vi "anschlüsse.vi"() -> ()   [LabVIEW 2010]
uses:
  <vilib>/numeric/LVNumericRepresentation.ctl
  <vilib>/Utility/miscctls.llb/LVPointTypeDef.ctl
panel:
  in  "poly2-Pfad":path
  in  "VI-Pfad":path
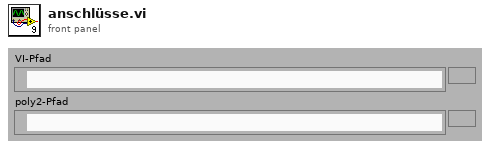
[diagram p1: front panel]
types:
  T1 = typedef "LVNumericRepresentation.ctl" = enum32{"Extended Precision", "Double Precision", "Single Precision", "Long", "Word", "Byte", "Unsigned Long", "Unsigned Word", "Unsigned Byte", "Complex Extended", "Complex Double", "Complex Single", "Quad", "Unsigned Quad", "Fixed-Point"}
  T2 = typedef "LVPointTypeDef.ctl" = cluster{"Horizontal":i16, "Vertical":i16}
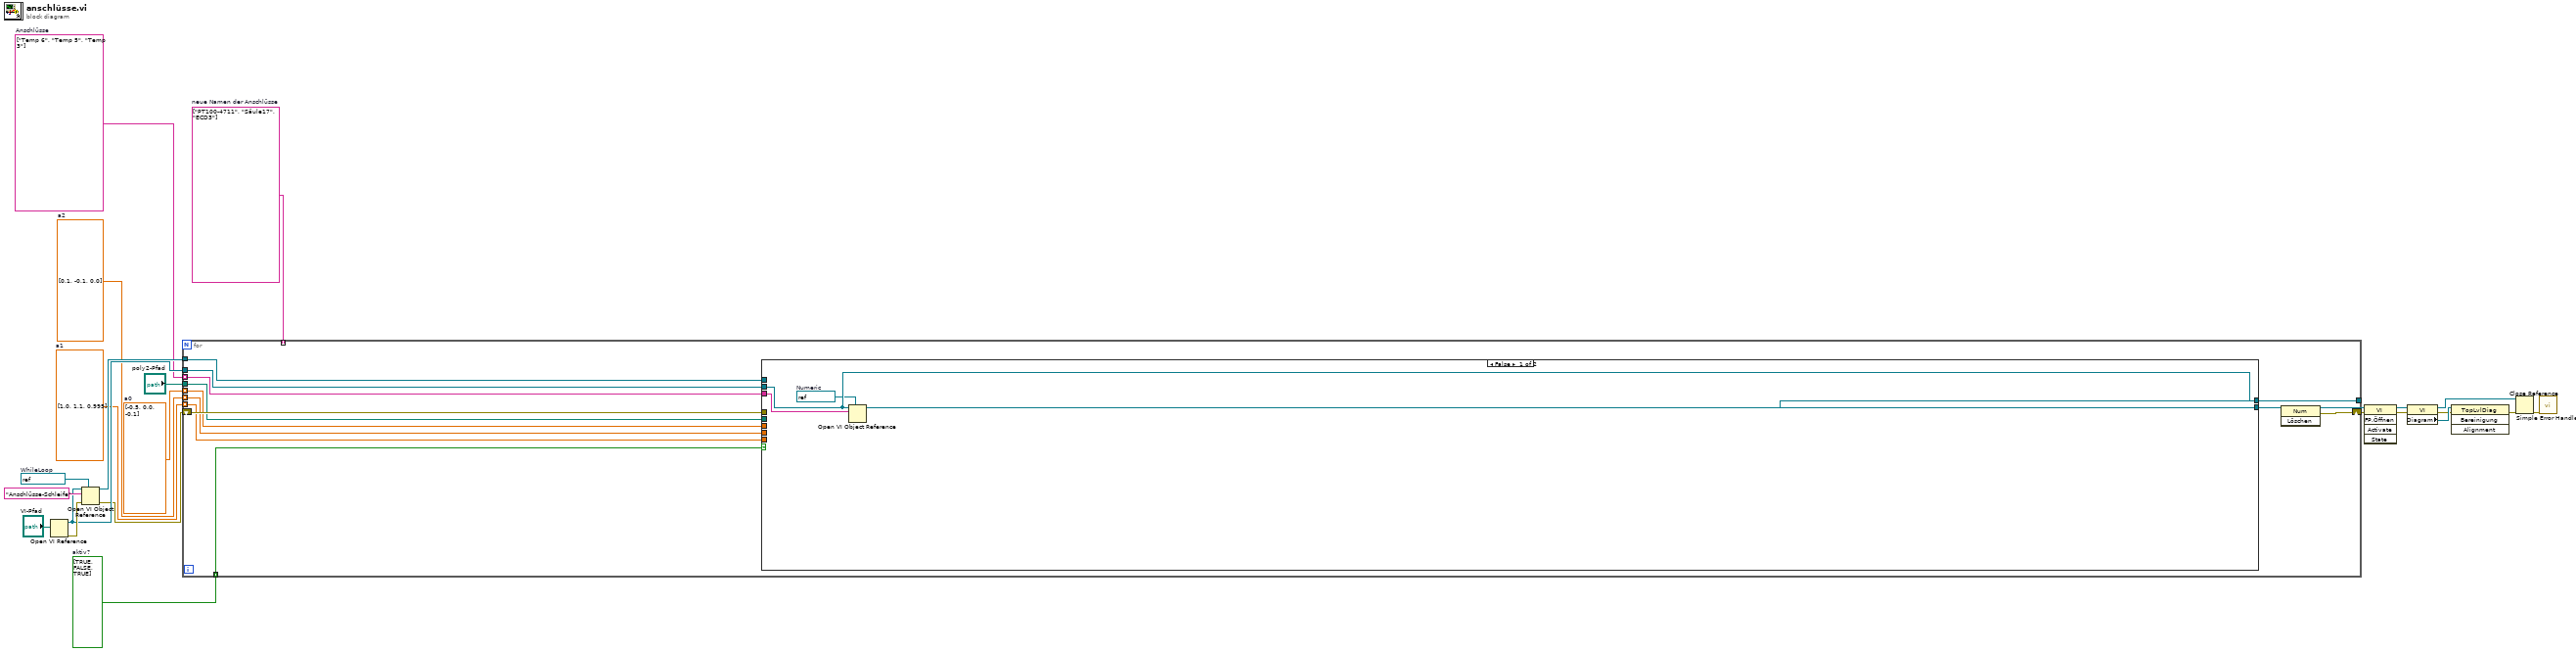
[diagram p0: block diagram]
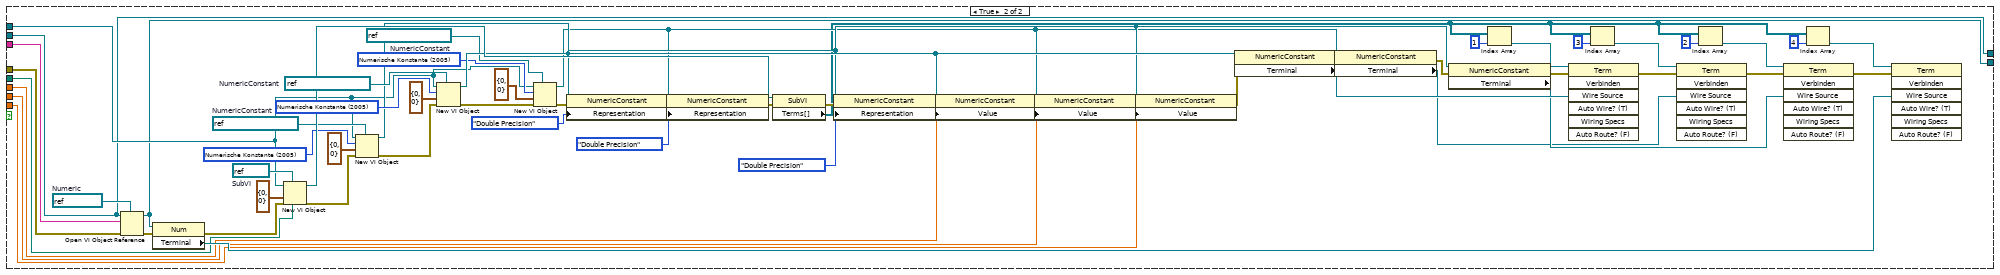
[diagram p2: hidden frame]
diagram:
  w1 = string[] ["PT100-4711", "Säule17", "ECD3"]  # neue Namen der Anschlüsse
  w2 = bool[] [TRUE, FALSE, TRUE]  # aktiv?
  w4 = dbl[] [-0.5, 0.0, -0.1]  # a0
  w5 = dbl[] [1.0, 1.1, 0.995]  # a1
  w6 = dbl[] [0.1, -0.1, 0.0]  # a2
  w15 = string[] ["Temp 6", "Temp 5", "Temp 3"]  # Anschlüsse
  w20 = refnum<vi> refnum  # WhileLoop
  n1 = Open VI Reference(vi path="VI-Pfad") -> (vi reference=w18:refnum<vi>, error out=w21:errorcluster)  [unwired: 5 in]
  n2 = Open VI Object Reference(7:w20, 8:w21, 10:"Anschlüsse-Schleife" ("Name/Position"), 11:w18) -> (0:w17:errorcluster, 3:w16:refnum<vi>)
  n3 = for {
    tunnel: w18 -> [w32]
    shift-right: [w35] -> w10
    shift-left: w17 -> [w34]
    tunnel: w16 -> [w33]
    tunnel: [w25] -> w3
    tunnel: w15 -> [w30] mode=indexing
    tunnel: "poly2-Pfad" -> [w31]
    tunnel: w6 -> [w28] mode=indexing
    tunnel: w5 -> [w27] mode=indexing
    tunnel: w4 -> [w29] mode=indexing
    tunnel: w2 -> [w24] mode=indexing
    tunnel: w1 -> [_] mode=indexing
    n4 = case shown="False" w24 {
      tunnel: w34 -> [_ w48]
      tunnel: w33 -> [_ w47]
      tunnel: w32 -> [w39 w40]
      tunnel: w31 -> [_ w46]
      tunnel: w30 -> [w38 w45]
      tunnel: w29 -> [_ w44]
      tunnel: w28 -> [_ w43]
      tunnel: w27 -> [_ w42]
      tunnel: [w36 w41] -> w26
      tunnel: [w39 w40] -> w25
      frame False {
        w37 = refnum<vi> refnum  # Numeric
        n5 = Open VI Object Reference(7:w37, 10:w38, 11:w39) -> (3:w36:refnum<vi>)  [unwired: 1 in, 1 out]
      }
      frame True {
        w77 = 2005 items=[".NET (Referenz)"=3441, ".NET-Container"=2125, "1D-Array dezimieren"=2046, "1D-Array durchsuchen"=1901, "1D-Array interpolieren"=1905, "1D-Array rotieren"=1906, "1D-Array sortieren"=1120, "1D-Array teilen"=1908, "1D-Array transponieren"=23068, "1D-Array umkehren"=1900, "1D-Arrays überführen"=2045, "2D-Array transponieren"=1902, "2D-Bild"=3508, "3-Zustands-Feld (System)"=21333, "3D-Bild"=23776, "Abbrechen-Schaltfläche (Modern)"=21739, "Abbrechen-Schaltfläche (System)"=3131, "Abgerundetes Rechteck"=3611, "Abgesenkter Kreis"=3604, "Abgesenkter Menüring"=3019, "Abgesenkter Rahmen (Modern)"=3607, "Abgesenkter Rahmen (System)"=3624, "Abgesenktes abgerundetes Rechteck"=3638, "Abgesenktes Dreieck (abwärts)"=3619, "Abgesenktes Dreieck (aufwärts)"=3618, "Abgesenktes Dreieck (links)"=3616, "Abgesenktes Dreieck (rechts)"=3617, "Abgesenktes Rechteck (dick)"=3635, "Abgesenktes Viereck"=3601, "Abgesenktes Viereck (abgerundet)"=3610, "Absoluter Wert"=1054, "ActiveX (Referenz)"=3410, "ActiveX-Container"=2072, "ActiveX-Objekt schließen"=8001, "ActiveX-Objekt öffnen"=8000, "Addieren"=1050, "AdrErstellen"=1967, "Agitator"=3831, "Aktivieren der Menüüberwachung"=9002, "AllSpoll"=1960, "Anzahl der Cache-Level"=24133, "Anzahl der Datensätze ermitteln"=8064, "Anzahl der Datensätze festlegen"=8075, "Applikationsreferenz"=3412, "Applikationsreferenz öffnen"=8012, "Arcuscosecans"=23050, "Arcuscosinus"=1207, "Arcuscotangens"=23052, "Arcussecans"=23051, "Arcussinus"=1206, "Arcustangens"=1208, "Arcustangens (2 Eingänge)"=1228, "Areacosecans"=23056, "Areacosinus Hyperbolicus"=1218, "Areacotangens"=23058, "Areasecans"=23057, "Areasinus Hyperbolicus"=1217, "Areatangens Hyperbolicus"=1219, "Array (Blockdiagrammkonstante)"=2070, "Array (Klassisch)"=3300, "Array (Modern)"=21608, "Array aus Strings nach Pfad"=1422, "Array erstellen"=2041, "Array indizieren"=2042, "Array initialisieren"=2053, "Array Interface Control"=23777, "Array nach Cluster"=1168, "Array nach Tabellen-String"=1540, "Array umformen"=2055, "Array wieder zusammensetzen"=2403, "Array zerlegen"=2412, "Array-Elemente addieren"=1903, "Array-Elemente multiplizieren"=1904, "Array-Größe"=1809, "Auf Aktion warten"=1722, "Auf Frontpanel-Aktivität warten"=1328, "Auf GPIB-RQS warten"=1952, "Auf Meldung mit Melderhistorie warten"=9131, "Auf Meldung von mehreren mit Melderhistorie warten"=9132, "Auf Meldung von mehreren warten"=9106, "Auf Meldung warten"=9105, "Auf nächste ganze Zahl runden"=1055, "Auf nächstgrößere Zahl runden"=1076, "Auf nächstkleinere Zahl runden"=1075, "Auf Occurrence warten"=1701, "Auf Stream-Status warten"=23809, "Auf Stream-Verknüpfung warten"=23799, "Aufruf über Referenz"=3901, "Aufrufkette"=1999, "Aufschlüsseln"=2048, "Aus Array entfernen"=3912, "Aus Binärdatei lesen"=8051, "Aus Textdatei lesen"=8070, "Aus XML zurückkonvertieren"=8401, "Ausdrucksknoten"=2201, "Austauscher"=3828, "Auswahlfeld (Klassisch)"=3117, "Auswahlfeld (Modern)"=21924, "Auswahlfeld (System)"=3132, "Auswahlfeld (System) 1"=21900, "Auswählen"=1516, "Avogadro-Konstante (1/mol)"=23520, "Basis des natürlichen Logarithmus"=23510, "Basiseinheiten umwandeln"=1079, "Baumstruktur (Klassisch)"=21819, "Baumstruktur (Modern)"=21793, "Baumstruktur (System)"=21794, "Bedingte Deaktivierungsstruktur"=2064, "Benutzerdef. Referenz"=3428, "Benutzerdef. Referenz-Tag (Blockdiagrammkonstante)"=3426, "Benutzerdef. Referenz-Tag (Klassisch)"=3429, "Benutzerdef. Referenz-Tag (Modern)"=21745, "Benutzerdef. Tag (Blockdiagrammkonstante)"=2114, "Benutzerdef. Tag (Klassisch)"=3329, "Benutzerdef. Tag (Modern)"=21749, "Benutzerdefiniertes Trace-Ereignis erzeugen"=2250, "Benutzerereignis erstellen"=2073, "Benutzerereignis erzeugen"=2074, "Benutzerereignis löschen"=2075, "Benutzerobjekt"=3506, "Berechtigungen ermitteln"=8065, "Berechtigungen festlegen"=8076, "Bereich"=2196, "Bereich sperren"=1411, "Beschriftete Schaltfläche (Rechteck)"=3123, "Beschriftete Schaltfläche (Rund)"=3122, "Beschriftete Schaltfläche (runde Ecken)"=3124, "Beschriftete Schaltfläche (runde Kanten)"=3125, "Beschriftung (Modern)"=21960, "Beschriftung (System)"=21961, "Bildlaufleiste (horizontal)"=21110, "Bildlaufleiste (vertikal)"=21111, "Bis zum nächsten Vielfachen von ms warten"=1327, "Bitpack nach Array"=3135, "Bluetooth - Auf Listener warten"=9147, "Bluetooth - Erkennung"=9152, "Bluetooth - Lesen"=9149, "Bluetooth - Listener erstellen"=9151, "Bluetooth - Netzwerkverbindung (Referenz)"=3468, "Bluetooth - Schreiben"=9150, "Bluetooth - Verbindung beenden"=9148, "Bluetooth - Verbindung herstellen"=9153, "Boolescher Wert nach (0,1)"=1167, "Boolesches Array nach Zahl"=1815, "Bruch-/Exponential-String nach Zahl"=1187, "Byte-Array nach String"=1609, "Bytes tauschen"=1162, "Bytestream-Datei (Referenz)"=3408, "Bündeln"=2049, "CAN-Kanal (Blockdiagrammkonstante)"=2124, "CAN-Kanal (Klassisch)"=3340, "CAN-Kanal (Modern)"=21817, "CAN-Kanal (System)"=21966, "CAN-Schnittstelle (Blockdiagrammkonstante)"=2123, "CAN-Schnittstelle (Klassisch)"=3339, "CAN-Schnittstelle (Modern)"=21815, "CAN-Schnittstelle (System)"=21964, "CAN-Task (Blockdiagrammkonstante)"=3471, "CAN-Task (Klassisch)"=3470, "CAN-Task (Modern)"=21789, "CAN-Task (System)"=21963, "Case-Struktur"=2001, "Cluster (Klassisch)"=3400, "Cluster (Modern)"=21607, "Cluster nach Array"=1169, "Cluster-Array erstellen"=2047, "Cluster-Array indizieren und bündeln"=2056, "Cluster-Konstante"=2071, "Code-Interface-Knoten"=2050, "Cosecans"=1204, "Cosecans Hyperbolicus"=23053, "Cosinus"=1201, "Cosinus Hyperbolicus"=1215, "Cotangens"=1205, "Cotangens Hyperbolicus"=23055, "CPU-Informationen"=24130, "DAQ-Kanal (Traditionell) (Blockdiagrammkonstante)"=2085, "DAQ-Kanal (Traditionell) (Klassisch)"=3320, "DAQ-Kanal (Traditionell) (Modern)"=21733, "DAQmx - Analog-Trigger-Quelle (Blockdiagrammkonstante)"=2119, "DAQmx - Analog-Trigger-Quelle (Klassisch)"=3336, "DAQmx - Analog-Trigger-Quelle (Modern)"=21774, "DAQmx - Analog-Trigger-Quelle (System)"=21951, "DAQmx - Globaler Kanal (Blockdiagrammkonstante)"=3430, "DAQmx - Globaler Kanal (Klassisch)"=3443, "DAQmx - Globaler Kanal (Modern)"=21770, "DAQmx - Globaler Kanal (System)"=21957, "DAQmx - Physikalischer Kanal (Blockdiagrammkonstante)"=2118, "DAQmx - Physikalischer Kanal (Klassisch)"=3335, "DAQmx - Physikalischer Kanal (Modern)"=21777, "DAQmx - Physikalischer Kanal (System)"=21954, "DAQmx-Anschluss (Blockdiagrammkonstante)"=2117, "DAQmx-Anschluss (Klassisch)"=3319, "DAQmx-Anschluss (Modern)"=21781, "DAQmx-Anschluss (System)"=21955, "DAQmx-Gerätename (Blockdiagrammkonstante)"=2093, "DAQmx-Gerätename (Klassisch)"=3318, "DAQmx-Gerätename (Modern)"=21773, "DAQmx-Gerätename (System)"=21950, "DAQmx-Skalierungsname (Blockdiagrammkonstante)"=2116, "DAQmx-Skalierungsname (Klassisch)"=3317, "DAQmx-Skalierungsname (Modern)"=21775, "DAQmx-Skalierungsname (System)"=21952, "DAQmx-Switch (Blockdiagrammkonstante)"=2121, "DAQmx-Switch (Klassisch)"=3337, "DAQmx-Switch (Modern)"=21776, "DAQmx-Switch (System)"=21953, "DAQmx-Task-Name (Blockdiagrammkonstante)"=3434, "DAQmx-Task-Name (Klassisch)"=3442, "DAQmx-Task-Name (Modern)"=21778, "DAQmx-Task-Name (System)"=21959, "DataSocket-Referenz"=3417, "DataSocket: Lesen"=1086, "DataSocket: Schließen"=1085, "DataSocket: Schreiben"=1087, "DataSocket: Öffnen"=1084, "Datei lesen"=1407, "Datei schließen"=8052, "Datei schließen (veraltet)"=1405, "Datei schreiben"=1408, "Datei öffnen"=1403, "Datei- und Programmtyp"=1434, "Datei- und Programmtyp ermitteln"=8066, "Datei- und Programmtyp festlegen"=8077, "Datei-/Verzeichnis-Info"=8082, "Datei-/Verzeichnis-Info (veraltet)"=1413, "Dateidialog"=8058, "Dateidialog (veraltet)"=8081, "Dateigröße ermitteln"=8063, "Dateigröße festlegen"=8074, "Dateipfad-Anzeigeelement (Klassisch)"=3204, "Dateipfad-Anzeigeelement (Modern)"=21731, "Dateipfad-Bedienelement (Klassisch)"=3203, "Dateipfad-Bedienelement (Modern)"=21730, "Dateipfad-Bedienelement (System)"=21922, "Dateiposition ermitteln"=8062, "Dateiposition festlegen"=8073, "Dateipuffer leeren"=8059, "Dateipuffer leeren (veraltet)"=1406, "Daten serialisieren"=1164, "Daten-Cache-Größe"=24132, "Datenprotokoll lesen"=8069, "Datenprotokoll schreiben"=8079, "Datenprotokolldatei (Referenz)"=3402, "Datenträger-Info"=1414, "Datenträger-Info lesen"=8067, "Datenwertreferenz löschen"=2409, "Datum-/Zeit-String lesen"=1600, "Datum/Zeit formatieren"=8100, "Datum/Zeit in Sekunden ermitteln"=1303, "Datum/Zeit nach Sekunden"=1308, "Dekrementieren"=1058, "DevClear"=1961, "DevClearList"=1962, "Dezimal-String nach Zahl"=1184, "Dezimalzeichen gleich?"=23064, "Dezimalziffer?"=1119, "Diagrammdeaktivierungsstruktur"=2054, "Dialogfeld mit einer Schaltfläche"=1340, "Dialogfeld mit zwei Schaltflächen"=1341, "Digitaldaten (Klassisch)"=3210, "Digitaldaten (Modern)"=21216, "Digitaler Signalverlaufsgraph (Klassisch)"=3511, "Digitaler Signalverlaufsgraph (Modern)"=21718, "Dividieren"=1053, "Dividieren (mit Fehleranschlüssen)"=3918, "Dlg Horiz. Bildlaufleiste"=21905, "Dlg Numerisch 1"=2100, "Dlg Numerisch 2"=3006, "Dlg String"=2110, "Dlg Vert. Bildlaufleiste"=21906, "Drehknopf (Klassisch)"=3005, "Drehknopf (Modern)"=21000, "Drehregler (Klassisch)"=3050, "Drehregler (Modern)"=21732, "Drehspulinstrument (Klassisch)"=3030, "Drehspulinstrument (Modern)"=21008, "Dreieck (abwärts)"=3623, "Dreieck (aufwärts)"=3622, "Dreieck (links)"=3620, "Dreieck (rechts)"=3621, "Dreiecksrelief (abwärts)"=3615, "Dreiecksrelief (aufwärts)"=3614, "Dreiecksrelief (links)"=3612, "Dreiecksrelief (rechts)"=3613, "Druckbar?"=1124, "Druckschalter"=21001, "Druckschalter (rechteckig)"=3119, "Druckschalter (rechteckig) (Profil)"=3113, "Druckschalter (rund)"=3118, "Druckschalter (rund) (Profil)"=3112, "Drucktank (flach)"=3075, "Drucktank (Klassisch)"=3070, "Drucktank (Modern)"=21751, "Drucktank (schattiert)"=21753, "Dynamische FPGA-Schnittstellen-Umwandlung"=5690, "Eigenschaftsknoten"=1920, "Ein Element aus Stream auslesen"=23797, "Ein Element in Stream schreiben"=23798, "Einfacher horiz. Schieber"=3003, "Einfacher String"=2115, "Einfacher vert. Schieber"=3002, "Einfaches numerisches Feld"=2900, "Einheit umrechnen"=2059, "Element am Anfang einfügen"=9129, "Element aus Queue entfernen"=9113, "Element einfügen"=9111, "Element einfügen (verlustbehaftet)"=9130, "Elementarladung (C)"=23517, "Elementreferenz"=3419, "Elternmethode aufrufen"=2354, "Empfangen"=1974, "Empfangsendpunkt für Netzwerk-Stream erstellen"=23811, "EnableLocal"=1963, "EnableRemote"=1964, "Enum (Klassisch)"=3023, "Enum (Modern)"=21605, "Enum (System)"=3062, "Enum-Konstante"=2090, "EOF"=1410, "Ereignis-Callback (Referenz)"=3435, "Ereignis-Callback registrieren"=2078, "Ereignisdatenknoten"=2102, "Ereignisregistrierung aufheben"=2076, "Ereignisstruktur"=2052, "Ersten String suchen"=1532, "Erster Aufruf?"=1083, "Exklusiv-NICHT-ODER"=1073, "Exklusiv-ODER"=1063, "Exponential"=1211, "Exponential (Arg) -1"=1222, "FALSE-Konstante"=2006, "Farbfeld"=3013, "Farbfeld mit dünnem Rahmen"=2905, "Farbfeld mit Rahmen (Klassisch)"=3008, "Farbfeld mit Rahmen (Modern)"=21019, "Farbfeldkonstante"=2120, "Farbiges Rechteck (Fehler?)"=3625, "Farbrampe"=3022, "Fehler zusammenfassen"=2147, "Fehler-Ringkonstante"=2039, "Festkomma in Integer umwandeln"=5566, "Festkomma-Überlaufzustand einschließen"=5564, "Festkomma-Überlaufzustand entfernen"=5563, "Festkomma-Überlaufzustand löschen"=5562, "Festkommakomponenten erfassen"=11163, "Festkommaüberlauf?"=5565, "FieldPoint-I/O-Kanal (Blockdiagrammkonstante)"=3440, "FieldPoint-I/O-Kanal (Klassisch)"=3439, "FieldPoint-I/O-Kanal (Modern)"=21784, "FIFO (Referenz)"=3474, "FindLstn"=1965, "FindRQS"=1966, "Flache Sequenzstruktur"=2069, "Fließkantenrelief (horizontal)"=3633, "Fließkantenrelief (vertikal)"=3634, "For-Schleife"=2002, "Formelknoten"=2004, "FPGA-Referenz nach Session"=2322, "Freie Beschriftung"=2321, "Frontpanel-Aktivität generieren"=1329, "Förderband"=3827, "Für Ereignisse registrieren"=2065, "Gabelung"=2194, "Gerät lesen"=1432, "Gerät schreiben"=1431, "Gerät öffnen"=1430, "Gerätereferenz"=3405, "Gerätsteuerung/Status"=1433, "Gestapelte Sequenzstruktur"=2000, "Gleich 0?"=1113, "Gleich?"=1102, "Globale Variable"=2060, "GPIB: Initialisierung"=1957, "GPIB: Lesen"=1951, "GPIB: Schreiben"=1950, "GPIB: Serielles Pollen"=1955, "GPIB: Status"=1959, "GPIB: Trigger"=1953, "GPIB: Verschiedenes"=1956, "GPIB: Warten"=1958, "GPIB: Zurücksetzen"=1954, "Grafikring (Klassisch)"=3015, "Grafikring (Modern)"=21602, "Grafikring (System)"=21925, "Gravitationskonstante (N m2/kg2)"=23519, "Größen-Handle"=1603, "Größer als 0?"=1117, "Größer oder gleich 0?"=1114, "Größer oder gleich?"=1103, "Größer?"=1110, "Heizkessel"=3829, "Hexadezimal-String nach Zahl"=1185, "Hexadezimalziffer?"=1123, "Hilfefenster steuern"=1353, "Hinzufügen (mit Fehleranschlüssen)"=3915, "Horiz. Linie"=3821, "Horiz. Rohrleitung (flach)"=3810, "Horiz. Rohrleitung (schattiert)"=3710, "Horiz. Rundbox"=3636, "Horizontaler Trennbalken (Klassisch)"=21863, "Horizontaler Trennbalken (System)"=21865, "ID des aktuellen Prozessors"=24131, "IMAQ-Session"=3415, "Immer kopieren"=2400, "Implikation"=1080, "In Array einfügen"=3911, "In Binärdatei schreiben"=8078, "In Datei formatieren"=2083, "In Datei suchen"=2082, "In Großbuchstaben"=1188, "In Kleinbuchstaben"=1189, "In OLE-Variant"=8002, "In String formatieren"=2081, "In String suchen"=2080, "In Textdatei schreiben"=8080, "In XML konvertieren"=8400, "Inkrementieren"=1057, "Inline-C-Knoten"=2104, "Inplace-Elementstruktur"=2360, "Integer in Festkomma umwandeln"=5567, "Intensitätsdiagramm (Klassisch)"=3509, "Intensitätsdiagramm (Modern)"=21719, "Intensitätsgraph (Klassisch)"=3510, "Intensitätsgraph (Modern)"=21720, "Intervall #1"=3073, "Intervall #2"=21755, "IP nach String"=1710, "IrDA-Netzwerkverbindung (Referenz)"=3450, "IrDA: Auf Listener warten"=9143, "IrDA: Geräte suchen"=9141, "IrDA: Lesen"=9145, "IrDA: Listener erzeugen"=9140, "IrDA: Schreiben"=9146, "IrDA: Verbindung herstellen"=9142, "IrDA: Verbindung schließen"=9144, "IVI Session löschen"=8103, "Kehrwert"=1059, "Kehrwert von e"=23511, "Kehrwert von Pi"=23507, "Kein Pfad (Konstante)"=23524, "Keine Referenz (Konstante)"=23526, "Keine Umgebungsvariable"=23527, "Keine Zahl/Kein Pfad/Keine Referenz?"=1128, "Kippschalter"=21002, "Kippschalter (vertikal)"=21740, "Klassenbezeichner-Konstante"=2094, "Kleiner als 0?"=1118, "Kleiner oder gleich 0?"=1115, "Kleiner oder gleich?"=1104, "Kleiner?"=1111, "Knoten zum Aufruf externer Bibliotheken"=2062, "Kombinationsfeld (Klassisch)"=3304, "Kombinationsfeld (Modern)"=21604, "Kombinationsfeld (System)"=21917, "Kombinationsfeldkonstante"=2088, "Komplex nach polar"=1045, "Komplex nach Re/Im"=1044, "Komplex-Konjugierte"=1048, "Kompressor"=3832, "Konstruktorknoten"=3904, "Kopieren"=8053, "Kopieren (veraltet)"=1416, "Kreis"=3605, "Kreisförmiges Relief"=3603, "Kreuzung"=2197, "LabVIEW beenden"=1352, "LabVIEW-Objekt"=3457, "Laufzeitklasse erhalten"=8018, "Leak Variant Value Reference"=2410, "LED (rechteckig) (Klassisch)"=3121, "LED (rechteckig) (Modern)"=21013, "LED (rund) (Klassisch)"=3120, "LED (rund) (Modern)"=21012, "LED-Schalter"=3116, "Leerer Pfad (Konstante)"=23523, "Leerer String (Konstante)"=23503, "Leerer String/Pfad?"=1112, "Leeres Array?"=23063, "Leuchte (rechteckig)"=3105, "Leuchte (rund)"=3104, "Lexikalische Klasse"=1126, "Lichtgeschwindigkeit im Vakuum (m/s)"=23518, "Linie (dick)"=3629, "Linie (dünn)"=3626, "Linie (vertieft) (System)"=3632, "Linie (vertieft, dick)"=3630, "Linie (vertieft, dünn)"=3627, "Linie mit Pfeil (dick)"=3631, "Linie mit Pfeil (dünn)"=3628, "Listenfeld (Klassisch)"=21806, "Listenfeld (Modern)"=21792, "Listenfeld (System)"=21805, "Listenfeldsymbol-Ringkonstante"=2038, "Logarithmus zur Basis 10"=1210, "Logarithmus zur Basis 10 von e"=23512, "Logarithmus zur Basis 2"=1225, "Logarithmus zur Basis x"=1224, "Logischer IVI-Name (Blockdiagrammkonstante)"=3420, "Logischer IVI-Name (Klassisch)"=3414, "Logischer IVI-Name (Modern)"=21736, "Logisches Verschieben"=1081, "Lokale Variable"=2061, "Löschen"=8056, "Löschen (veraltet)"=1417, "Mantisse und Exponent"=1150, "Maschinengenauigkeit"=23528, "MathScript-Aufruf über Referenzknoten"=3906, "MathScript-Knoten"=2357, "MATLAB-Skript"=9020, "Matrix entpacken"=23000, "Matrix erstellen"=8500, "Matrix transponieren"=8509, "Matrixdiagonale festlegen"=8504, "Matrixdiagonale lesen"=8501, "Matrixelemente festlegen"=8505, "Matrixelemente lesen"=8502, "Matrixgröße"=8507, "Matrixgröße ändern"=8508, "Max & Min"=1108, "Max. & Min. von Array"=1907, "Mehrere Elemente aus Stream auslesen"=23803, "Mehrere Elemente in Stream schreiben"=23804, "Mehrfacharithmetik"=2200, "Mehrsegmentrohr"=23780, "Mehrspaltiges Listenfeld (Klassisch)"=21799, "Mehrspaltiges Listenfeld (Modern)"=21791, "Mehrspaltiges Listenfeld (System)"=21798, "Melder anfordern"=9101, "Melder freigeben"=9102, "Melderreferenz"=3423, "Melderstatus lesen"=9103, "Meldung abbrechen"=9107, "Meldung senden"=9104, "Menü-Popup-Ring"=3017, "Menüauswahl abfragen"=9001, "Menüleiste des aktuellen VIs"=9000, "Menüpunkt-Info lesen"=9005, "Menüpunkte einfügen"=9003, "Menüpunkte löschen"=9004, "Menüpunkteinstellungen"=9006, "Menüreferenz"=3413, "Menüring (Klassisch)"=3018, "Menüring (Modern)"=21600, "Menüverknüpfung abfragen"=9007, "Messleiste (horizontal)"=21106, "Messleiste (vertikal)"=21107, "Methodenknoten"=3900, "Mischsignalgraph"=21721, "Mit Potenz von 2 multiplizieren"=1074, "Molare Gas-Konstante (J/(mol K))"=23522, "Motion-Ressource (Blockdiagrammkonstante)"=3449, "Motion-Ressource (Klassisch)"=3448, "Motion-Ressource (Modern)"=21787, "Motor (flach)"=3820, "Motor (schattiert)"=3720, "Multifrequenzstruktur"=2199, "Multiplizieren"=1052, "Multiplizieren (mit Fehleranschlüssen)"=3917, "Muster suchen"=1535, "Nach allgemeinerer Klasse"=8017, "Nach Byte-Integer"=1140, "Nach Festkomma"=5561, "Nach Fließkommawert (doppelte Genauigkeit)"=1147, "Nach Fließkommawert (einfache Genauigkeit)"=1146, "Nach Fließkommawert (erweitert)"=1149, "Nach Komplex (doppelte Genauigkeit)"=1152, "Nach Komplex (einfache Genauigkeit)"=1151, "Nach Komplex (höchste Genauigkeit)"=1154, "Nach links rotieren (mit Übertrag)"=1606, "Nach Long-Integer"=1142, "Nach Namen aufschlüsseln"=2058, "Nach Namen bündeln"=2057, "Nach Quad-Integer"=1155, "Nach rechts rotieren (mit Übertrag)"=1607, "Nach Sonden-String"=2413, "Nach spezifischerer Klasse"=8016, "Nach Variant"=8201, "Nach vorzeichenlosen Byte-Integer"=1143, "Nach vorzeichenlosen Long-Integer"=1145, "Nach vorzeichenlosen Quad-Integer"=1156, "Nach vorzeichenlosen Wort-Integer"=1144, "Nach Wert durchsuchen"=1534, "Nach Wort-Integer"=1141, "Nach Zeitstempel"=5560, "Natürlicher Logarithmus"=1209, "Natürlicher Logarithmus (Arg +1)"=1221, "Natürlicher Logarithmus von 10"=23513, "Natürlicher Logarithmus von 2"=23514, "Natürlicher Logarithmus von Pi"=23508, "Negativ unendlich"=23509, "Negieren"=1069, "Neue Datei"=1404, "Neue Datenwertreferenz"=2408, "Neue IVI-Session"=8102, "Neues Verzeichnis"=1402, "Neues VI"=8014, "Neues VI-Objekt"=8015, "NICHT"=1064, "Nicht darstellbares Zeichen?"=1125, "Nicht-ODER"=1072, "Nicht-UND"=1071, "Numerische Konstante"=2005, "Numerisches Anzeigeelement (Klassisch)"=3001, "Numerisches Anzeigeelement (Modern)"=21004, "Numerisches Bedienelement (Klassisch)"=3000, "Numerisches Bedienelement (Modern)"=21003, "Numerisches Bedienelement (System)"=21919, "Occurrence (Referenz)"=3406, "Occurrence erzeugen"=1700, "Occurrence festlegen"=1702, "ODER"=1062, "ODER (Array-Elemente)"=1910, "Offener Tank (flach) (Klassisch)"=21752, "Offener Tank (schattiert) (Klassisch)"=3074, "OK-Schaltfläche (Modern)"=21738, "OK-Schaltfläche (System)"=3130, "Oktal-String nach Zahl"=1186, "Oktalziffer?"=1129, "OLE-Variant"=3150, "Online-Hilfe steuern"=1355, "Optionsfeld (rechteckig)"=3107, "Optionsfeld (rund)"=3106, "Optionsfeld (System)"=3133, "Optionsfelder (Klassisch)"=22003, "Optionsfelder (Modern)"=22001, "Optionsfelder (System)"=22002, "Ordner anzeigen"=8083, "Ordner erstellen"=8055, "Paketmatrix"=23001, "PassControl"=1968, "Peek-Operation verarbeiten"=1604, "Pfad des aktuellen VIs"=1426, "Pfad erstellen"=1419, "Pfad nach Array aus Strings"=1423, "Pfad nach String"=1077, "Pfad zerlegen"=1420, "Pfadkonstante"=2009, "Pfadtyp"=1421, "Pfeil (Abwärts)"=3824, "Pfeil (aufwärts)"=3823, "Pfeil (links)"=3826, "Pfeil (rechts)"=3825, "Pi"=23504, "Pi geteilt durch 2"=23506, "Pi multipliziert mit 2"=23505, "PixMap"=3505, "PixMap (Warnung: gefährlich)"=3507, "Planck-Konstante (J/Hz)"=23516, "Plattform: Flache Rechteck-Schaltfläche"=3134, "Plugin-Steuerung"=21820, "Poke-Operation verarbeiten"=1605, "Polar nach komplex"=1047, "Polar nach Re/Im"=23061, "Position im Datenprotokoll ermitteln"=8061, "Position im Datenprotokoll festlegen"=8072, "Positiv unendlich"=23515, "Potenz von 10"=1212, "Potenz von 2"=1223, "PPoll"=1969, "PPollConfig"=1970, "PPollUnconfig"=1971, "Pulldown-Menüring"=3061, "Pumpe (links) (flach)"=3813, "Pumpe (links) (schattiert)"=3713, "Pumpe (rechts) (flach)"=3819, "Pumpe (rechts) (schattiert)"=3719, "Quadrat"=23059, "Quadratwurzel"=1060, "Queue anfordern"=9108, "Queue freigeben"=9109, "Queue leeren"=9114, "Queue-Referenz"=3424, "Queue-Status lesen"=9110, "Quotient und Rest"=1056, "Rahmen"=3608, "RcvRespMsg"=1972, "Re/Im nach komplex"=1046, "Re/Im nach polar"=23060, "ReadStatus"=1973, "ReceiveSetup"=1975, "Rechteck"=3602, "Rechteckschaltfläche"=3103, "Referenz nach Pfad"=1424, "Referenz nach Session"=2306, "Referenz schließen"=8011, "Regel- und Simulationsschleife"=2099, "Registerkartenelement (Klassisch)"=3330, "Registerkartenelement (Modern)"=3332, "Registerkartenelement (System)"=3331, "Registrierung für Sitzung entfernen"=2320, "Registrierungssession"=2319, "Reliefrahmen"=3606, "ResetSys"=1976, "Ressourcen-Index"=1088, "Rohrknie (links, abwärts) (flach)"=3811, "Rohrknie (links, abwärts) (schattiert)"=3711, "Rohrknie (links, aufwärts) (flach)"=3708, "Rohrknie (links, aufwärts) (flach) 1"=3808, "Rohrknie (rechts, abwärts) (flach)"=3817, "Rohrknie (rechts, abwärts) (schattiert)"=3717, "Rohrknie (rechts, aufwärts) (flach)"=3814, "Rohrknie (rechts, aufwärts) (schattiert)"=3714, "Rotationsverteiler"=3830, "Rotieren"=1082, "RT-FIFO erstellen"=24000, "RT-FIFO lesen"=24001, "RT-FIFO löschen"=24003, "RT-FIFO schreiben"=24002, "Rundinstrument (Klassisch)"=3040, "Rundinstrument (Modern)"=21009, "Rundschaltfläche"=3102, "Rydberg-Konstante (1/m)"=23521, "Rückkopplungsknoten"=2353, "Schalter (horizontal)"=3108, "Schalter (vertikal)"=3109, "Schaltfläche (rechteckig)"=3101, "Schaltfläche (rund)"=3100, "Schieber (horizontal) (Klassisch)"=3010, "Schieber (horizontal) (System)"=21904, "Schieber (horizontal, gefüllt) (Klassisch)"=3012, "Schieber (horizontal, gefüllt) (Modern)"=21100, "Schieber (vertikal) (System)"=21903, "Schieber (vertikal, gefüllt) (Klassisch)"=3009, "Schieber (vertikal, gefüllt) (Modern)"=21014, "Schieber mit Knopf (vertikal)"=3004, "Schieber mit Zeiger (horizontal) (Klassisch)"=3011, "Schieber mit Zeiger (horizontal) (Modern)"=21101, "Schieber mit Zeiger (horizontal) (System)"=21902, "Schieber mit Zeiger (vertikal) (Klassisch)"=3007, "Schieber mit Zeiger (vertikal) (Modern)"=21017, "Schieber mit Zeiger (vertikal) (System)"=21901, "Schiebeschalter"=21011, "Schiebeschalter (horizontal)"=3114, "Schiebeschalter (vertikal) (Klassisch)"=3115, "Schiebeschalter (vertikal) (Modern)"=21741, "Schwellwert (1D-Array)"=1909, "Secans"=1203, "Secans Hyperbolicus"=23054, "Sekunden nach Datum/Zeit"=1309, "SendCmds"=1978, "SendDataBytes"=1979, "Sendeendpunkt für Netzwerk-Stream erstellen"=23810, "Senden"=1977, "SendIFC"=1980, "SendList"=1981, "SendLLO"=1982, "SendSetup"=1983, "Serialisierte Daten nach Variant"=8202, "Serialisiertes benutzerdef. Referenz-Tag (Klassisch)"=3454, "Serialisiertes benutzerdef. Referenz-Tag (Modern)"=21747, "Session nach Referenz"=2307, "SetRWLS"=1984, "SetTimeOut"=1985, "Signale trennen"=2351, "Signale zusammenfassen"=2350, "Signalverlauf erstellen"=2066, "Signalverlaufsattribut entfernen"=8209, "Signalverlaufsattribut ermitteln"=8208, "Signalverlaufsattribut festlegen"=8207, "Signalverlaufsdiagramm"=21010, "Signalverlaufsdiagramm (Klassisch)"=3501, "Signalverlaufsdiagramm (Modern)"=21717, "Signalverlaufsgraph (Klassisch)"=3504, "Signalverlaufsgraph (Modern)"=21703, "Signalverlaufskomponenten lesen"=2067, "Sinc"=1227, "Sinus"=1200, "Sinus Hyperbolicus"=1214, "Sinus und Cosinus"=1220, "Speicherfreigabe anfordern"=1610, "Standardverzeichnis"=1427, "Statische VI-Referenz"=2084, "Status des Hilfefensters lesen"=1354, "Stopp"=1350, "Stopp-Schaltfläche"=21230, "Stopp-Schaltfläche (rechteckig)"=3128, "Stopp-Schaltfläche (rund)"=3127, "Stream beenden"=23807, "Stream erstellen"=23796, "Stream leeren"=23808, "Stream prüfen und verknüpfen"=23805, "Stream starten"=23806, "Stream verknüpfen"=23793, "Stream-Endpunkt entfernen"=23794, "Stream-Verknüpfung aufheben"=23795, "String deserialisieren"=1165, "String durchsuchen und teilen"=1538, "String nach Byte-Array"=1608, "String nach IP"=1711, "String nach Pfad"=1078, "String nach Token durchsuchen"=8101, "String nach Umgebungsvariable"=1830, "String rotieren"=1536, "String suchen und ersetzen"=3914, "String umkehren"=1537, "String-Anzeigeelement (Klassisch)"=3201, "String-Anzeigeelement (Modern)"=21702, "String-Array indizieren"=1531, "String-Bedienelement (Klassisch)"=3200, "String-Bedienelement (Modern)"=21701, "String-Bedienelement (System)"=21920, "String-Konstante"=2007, "String-Länge"=1502, "Stringarray sortieren"=23065, "Strings verknüpfen"=2040, "Subtrahieren"=1051, "Subtrahieren (mit Fehleranschlüssen)"=3916, "Suchen"=1409, "T-Stück (abwärts) (flach)"=3818, "T-Stück (abwärts) (schattiert)"=3718, "T-Stück (aufwärts) (flach)"=3812, "T-Stück (aufwärts) (schattiert)"=3712, "T-Stück (links) (flach)"=3809, "T-Stück (links) (schattiert)"=3709, "T-Stück (rechts) (flach)"=3815, "T-Stück (rechts) (schattiert)"=3715, "Tabelle (Klassisch)"=21796, "Tabelle (Modern)"=21790, "Tabelle (System)"=21797, "Tabellen-String nach Array"=1539, "Tabulatorkonstante"=23502, "Tag-Attributring"=2063, "Tangens"=1202, "Tangens Hyperbolicus"=1216, "Tank (horizontal)"=3071, "Tank (Klassisch)"=3020, "Tank (Modern)"=21006, "TCP-Netzwerkverbindung (Referenz)"=3407, "TCP: Auf Listener warten"=1712, "TCP: Lesen"=1716, "TCP: Lesen (Flex.)"=1720, "TCP: Lesen (Strings)"=1718, "TCP: Listener erstellen"=1717, "TCP: Schreiben"=1714, "TCP: Schreiben (Flex.)"=1721, "TCP: Schreiben (Strings)"=1719, "TCP: Verbindung herstellen"=1715, "TCP: Verbindung schließen"=1713, "TDMS Close"=24113, "TDMS Defragment"=24119, "TDMS Flush"=24117, "TDMS Get Properties"=24115, "TDMS List Contents"=24116, "TDMS Open"=24112, "TDMS Read"=24111, "TDMS Refnum To File ID"=24120, "TDMS Set Properties"=24114, "TDMS Write"=24110, "TDMS Write IP"=24118, "TDMS: Datei"=3477, "Teil-Array"=2044, "Teil-Array ersetzen"=3910, "Teil-String"=1503, "Teil-String ersetzen"=3913, "Temporäres Verzeichnis"=1435, "TestSRQ"=1986, "TestSys"=1987, "Text nach UTF-8"=23066, "Text- & Grafikring (Klassisch)"=3016, "Text- & Grafikring (Modern)"=21603, "Text-Schaltfläche"=21015, "Textring (Blockdiagrammkonstante)"=2008, "Textring (Klassisch)"=3014, "Textring (Modern)"=21601, "Textring (System)"=3060, "Thermometer (Klassisch)"=3021, "Thermometer (Modern)"=21007, "Timer-Wert (ms)"=1300, "Trennbalken (horizontal)"=21861, "Trennbalken (vertikal)"=21860, "Trennschalter"=21020, "Trichter 1"=21754, "Trichter 2"=3072, "Trigger"=1988, "TriggerList"=1989, "TRUE/FALSE-String anhängen"=1511, "TRUE/FALSE-String suchen"=1533, "Typ erzwingen"=2402, "Typumwandlung"=1166, "UDP-Netzwerkverbindung (Referenz)"=3418, "UDP: Lesen"=1724, "UDP: Multicast öffnen"=1727, "UDP: Schließen"=1726, "UDP: Schreiben"=1725, "UDP: Öffnen"=1723, "Umgebungsvariable"=23778, "Umgebungsvariable nach String"=1831, "Umgebungsvariablenelement (Klassisch)"=3472, "Umgebungsvariablenelement (Modern)"=21814, "Umgebungsvariablenkonstante"=3473, "Umschalter (horizontal) (Klassisch)"=3110, "Umschalter (horizontal) (Modern)"=21700, "Umschalter (vertikal) (Klassisch)"=3111, "Umschalter (vertikal) (Modern)"=21005, "Unbitpack von Array"=3136, "UND"=1061, "UND (Array-Elemente)"=1911, "Ungleich 0?"=1116, "Ungleich?"=1105, "Unleak Variant Value Reference"=2411, "Untermatrix festlegen"=8506, "Untermatrix lesen"=8503, "Unterpanel"=21810, "Unterpanel (klassisch)"=21811, "Unterpanel (System)"=21823, "UTF-8 nach Text"=23067, "Variable auslesen (mit Timeout)"=23786, "Variable direkt lesen"=23785, "Variable direkt schreiben"=23788, "Variable lesen"=23781, "Variable lesen (Scan)"=23784, "Variable schreiben"=23782, "Variable schreiben (mit Timeout)"=23789, "Variable schreiben (Scan)"=23787, "Variablen-Container suchen"=23802, "Variablenklassenbezeichner-Konstante"=2106, "Variablenkonfiguration"=3475, "Variablenname (Konstante)"=3478, "Variablenverbindung beenden"=23783, "Variablenverbindung herstellen"=23779, "Variablenverbindung herstellen und prüfen"=23790, "Variablenverbindung im Hintergrund herstellen"=23791, "Variant"=3310, "Variant nach Daten"=8003, "Variant nach serialisierte Daten"=8203, "Variant wieder zusammensetzen (Warnung: gefährlich)"=2405, "Variant zerlegen"=2404, "Variantattribut entfernen"=8206, "Variantattribut ermitteln"=8205, "Variantattribut festlegen"=8204, "Vektorwerte austauschen"=1912, "Ventil (Abwärtsbogen) (flach)"=3707, "Ventil (Abwärtsbogen) (schattiert)"=21767, "Ventil (Abwärtsbogen) (Umriss)"=3807, "Ventil (Aufwärtsbogen) (flach)"=3703, "Ventil (Aufwärtsbogen) (schattiert)"=21763, "Ventil (Aufwärtsbogen) (Umriss)"=3803, "Ventil (Linksbogen) (flach)"=3701, "Ventil (Linksbogen) (schattiert)"=21761, "Ventil (Linksbogen) (Umriss)"=3801, "Ventil (Rechtsbogen) (flach)"=3705, "Ventil (Rechtsbogen) (schattiert)"=21765, "Ventil (Rechtsbogen) (Umriss)"=3805, "Ventil (rechtwinklig, abwärts) (flach)"=3706, "Ventil (rechtwinklig, abwärts) (schattiert)"=21766, "Ventil (rechtwinklig, abwärts) (Umriss)"=3806, "Ventil (rechtwinklig, aufwärts) (flach)"=3702, "Ventil (rechtwinklig, aufwärts) (schattiert)"=3802, "Ventil (rechtwinklig, aufwärts) (Umriss)"=21762, "Ventil (rechtwinklig, links) (flach)"=3700, "Ventil (rechtwinklig, links) (schattiert)"=21760, "Ventil (rechtwinklig, links) (Umriss)"=3800, "Ventil (rechtwinklig, rechts) (flach)"=3704, "Ventil (rechtwinklig, rechts) (schattiert)"=21764, "Ventil (rechtwinklig, rechts) (Umriss)"=3804, "Ventil prüfen"=3833, "Vereinigung"=2195, "Verlaufsanzeige (horizontal) (Modern)"=21102, "Verlaufsanzeige (horizontal) (System)"=21910, "Verlaufsanzeige (vertikal) (Modern)"=21104, "Verlaufsanzeige (vertikal) (System)"=21909, "Verschieben"=8068, "Verschieben (veraltet)"=1415, "Verschobene Daten ermitteln"=9154, "Vert. Linie"=3822, "Vert. Rohrleitung (flach)"=3816, "Vert. Rohrleitung (schattiert)"=3716, "Vertikaler Trennbalken (Klassisch)"=21862, "Vertikaler Trennbalken (System)"=21864, "Verzeichnis auflisten"=1418, "VI-Bibliothek"=1425, "VI-Objektreferenz öffnen"=8013, "VI-Referenz"=3422, "VI-Referenz öffnen"=8010, "VI-Server-Referenz"=2091, "Viereckiges Relief (Klassisch)"=3600, "Viereckiges Relief (Modern)"=3637, "Viereckiges Relief (runde Ecken)"=3609, "VISA-Referenz nach Session"=2300, "VISA-Ressourcenname"=3421, "VISA-Ressourcenname (Klassisch)"=3409, "VISA-Ressourcenname (Modern)"=21737, "VISA: Adresse freigeben"=1933, "VISA: Adresse zuweisen"=1932, "VISA: Auf Ereignis warten"=1943, "VISA: Bereich lesen (16)"=1948, "VISA: Bereich lesen (32)"=1991, "VISA: Bereich lesen (64)"=2144, "VISA: Bereich lesen (8)"=1946, "VISA: Bereich schreiben (16)"=1949, "VISA: Bereich schreiben (32)"=1992, "VISA: Bereich schreiben (64)"=2145, "VISA: Bereich schreiben (8)"=1947, "VISA: Ereignis aktivieren"=1942, "VISA: Ereignis deaktivieren"=1940, "VISA: Ereignis verwerfen"=1941, "VISA: GPIB sendet IFC"=2318, "VISA: GPIB steuert ATN"=2316, "VISA: GPIB steuert REN"=2304, "VISA: GPIB-Befehl"=2315, "VISA: GPIB-Durchgangssteuerung"=2317, "VISA: Hilfssignal anfordern"=2310, "VISA: I/O-Puffer entleeren"=2302, "VISA: I/O-Puffergröße festlegen"=2301, "VISA: In Datei lesen"=2313, "VISA: Interrupt anfordern"=2309, "VISA: Lesen"=1925, "VISA: Peek (16)"=1934, "VISA: Peek (32)"=1995, "VISA: Peek (64)"=2142, "VISA: Peek (8)"=1938, "VISA: Poke (16)"=1935, "VISA: Poke (32)"=1996, "VISA: Poke (64)"=2143, "VISA: Poke (8)"=1939, "VISA: Ressource suchen"=1923, "VISA: Schließen"=1922, "VISA: Schreiben"=1926, "VISA: Speicher freigeben"=1998, "VISA: Speicher reservieren"=1997, "VISA: Speicher reservieren (Ex)"=2146, "VISA: Sperre aufheben"=1994, "VISA: Sperren"=1993, "VISA: Statusinformation"=1924, "VISA: STB lesen"=1928, "VISA: Trigger freigeben"=2312, "VISA: Trigger freigeben 1"=1929, "VISA: Trigger zuweisen"=2311, "VISA: USB-Steuerung (Ausgang)"=2087, "VISA: USB-Steuerung (Eingang)"=2086, "VISA: Verschieben"=2303, "VISA: Von Datei schreiben"=2314, "VISA: VXI-Befehl oder -Abfrage"=2305, "VISA: Wert lesen (16)"=1930, "VISA: Wert lesen (32)"=1944, "VISA: Wert lesen (64)"=2140, "VISA: Wert lesen (8)"=1936, "VISA: Wert schreiben (16)"=1931, "VISA: Wert schreiben (32)"=1945, "VISA: Wert schreiben (64)"=2141, "VISA: Wert schreiben (8)"=1937, "VISA: Zurücksetzen"=1927, "VISA: Öffnen"=2308, "VISA: Öffnen (alt)"=1921, "Vorschau für Queue-Element"=9112, "Vorzeichen"=1049, "Wagenrücklauf-Konstante"=23500, "WaitSRQ"=1990, "Warten (ms)"=1302, "Wert formatieren"=1512, "Werte austauschen"=2401, "Wertebereich prüfen und erzwingen"=1127, "While-Schleife 1"=2003, "While-Schleife 2"=2352, "Words tauschen"=1163, "X hoch Y"=1213, "XY-Graph (Klassisch)"=3500, "XY-Graph (Modern)"=21716, "Y-te Wurzel von X"=23062, "Zahl nach boolesches Array"=1814, "Zahl nach Hexadezimal-String"=1181, "Zahl nach Oktal-String"=1182, "Zahl nach String (Dezimaldarstellung)"=1180, "Zahl nach String (Exponentialdarstellung)"=1505, "Zahl nach String (Fließkommadarstellung)"=1506, "Zahl nach String (Technische Notation)"=1183, "Zahl teilen"=1170, "Zahlen verbinden"=1171, "Zeile auswählen"=1510, "Zeilenende-Konstante"=23525, "Zeilenvorschub-Konstante"=23501, "Zeitgesteuerte Schleife"=5570, "Zeitgesteuerte Sequenz"=5573, "Zeitstempel (Blockdiagrammkonstante)"=2068, "Zeitstempel-Anzeigeelement (Klassisch)"=5556, "Zeitstempel-Anzeigeelement (Modern)"=21914, "Zeitstempel-Bedienelement (Klassisch)"=5555, "Zeitstempel-Bedienelement (modern)"=21913, "Zeitstempel-Bedienelement (System)"=21967, "ZerlegenGesperrteDatenWertRef"=2406, "Zufallszahl (0-1)"=1070, "Zugriff verweigern"=8057, "Zugriffsrechte"=1412, "ZusammensetzenSperreAufhebenDatenWertRef (Warnung: gefährlich)"=2407, "Zustand"=2198, "Zustandsdiagramm"=2051, "Öffnen/Erstellen/Ersetzen einer Datei"=8050, "Öffnen/Erstellen/Ersetzen einer Protokolldatei"=8054]
        w76 = refnum<vi> refnum  # NumericConstant
        w71 = 2005 items=[".NET (Referenz)"=3441, ".NET-Container"=2125, "1D-Array dezimieren"=2046, "1D-Array durchsuchen"=1901, "1D-Array interpolieren"=1905, "1D-Array rotieren"=1906, "1D-Array sortieren"=1120, "1D-Array teilen"=1908, "1D-Array transponieren"=23068, "1D-Array umkehren"=1900, "1D-Arrays überführen"=2045, "2D-Array transponieren"=1902, "2D-Bild"=3508, "3-Zustands-Feld (System)"=21333, "3D-Bild"=23776, "Abbrechen-Schaltfläche (Modern)"=21739, "Abbrechen-Schaltfläche (System)"=3131, "Abgerundetes Rechteck"=3611, "Abgesenkter Kreis"=3604, "Abgesenkter Menüring"=3019, "Abgesenkter Rahmen (Modern)"=3607, "Abgesenkter Rahmen (System)"=3624, "Abgesenktes abgerundetes Rechteck"=3638, "Abgesenktes Dreieck (abwärts)"=3619, "Abgesenktes Dreieck (aufwärts)"=3618, "Abgesenktes Dreieck (links)"=3616, "Abgesenktes Dreieck (rechts)"=3617, "Abgesenktes Rechteck (dick)"=3635, "Abgesenktes Viereck"=3601, "Abgesenktes Viereck (abgerundet)"=3610, "Absoluter Wert"=1054, "ActiveX (Referenz)"=3410, "ActiveX-Container"=2072, "ActiveX-Objekt schließen"=8001, "ActiveX-Objekt öffnen"=8000, "Addieren"=1050, "AdrErstellen"=1967, "Agitator"=3831, "Aktivieren der Menüüberwachung"=9002, "AllSpoll"=1960, "Anzahl der Cache-Level"=24133, "Anzahl der Datensätze ermitteln"=8064, "Anzahl der Datensätze festlegen"=8075, "Applikationsreferenz"=3412, "Applikationsreferenz öffnen"=8012, "Arcuscosecans"=23050, "Arcuscosinus"=1207, "Arcuscotangens"=23052, "Arcussecans"=23051, "Arcussinus"=1206, "Arcustangens"=1208, "Arcustangens (2 Eingänge)"=1228, "Areacosecans"=23056, "Areacosinus Hyperbolicus"=1218, "Areacotangens"=23058, "Areasecans"=23057, "Areasinus Hyperbolicus"=1217, "Areatangens Hyperbolicus"=1219, "Array (Blockdiagrammkonstante)"=2070, "Array (Klassisch)"=3300, "Array (Modern)"=21608, "Array aus Strings nach Pfad"=1422, "Array erstellen"=2041, "Array indizieren"=2042, "Array initialisieren"=2053, "Array Interface Control"=23777, "Array nach Cluster"=1168, "Array nach Tabellen-String"=1540, "Array umformen"=2055, "Array wieder zusammensetzen"=2403, "Array zerlegen"=2412, "Array-Elemente addieren"=1903, "Array-Elemente multiplizieren"=1904, "Array-Größe"=1809, "Auf Aktion warten"=1722, "Auf Frontpanel-Aktivität warten"=1328, "Auf GPIB-RQS warten"=1952, "Auf Meldung mit Melderhistorie warten"=9131, "Auf Meldung von mehreren mit Melderhistorie warten"=9132, "Auf Meldung von mehreren warten"=9106, "Auf Meldung warten"=9105, "Auf nächste ganze Zahl runden"=1055, "Auf nächstgrößere Zahl runden"=1076, "Auf nächstkleinere Zahl runden"=1075, "Auf Occurrence warten"=1701, "Auf Stream-Status warten"=23809, "Auf Stream-Verknüpfung warten"=23799, "Aufruf über Referenz"=3901, "Aufrufkette"=1999, "Aufschlüsseln"=2048, "Aus Array entfernen"=3912, "Aus Binärdatei lesen"=8051, "Aus Textdatei lesen"=8070, "Aus XML zurückkonvertieren"=8401, "Ausdrucksknoten"=2201, "Austauscher"=3828, "Auswahlfeld (Klassisch)"=3117, "Auswahlfeld (Modern)"=21924, "Auswahlfeld (System)"=3132, "Auswahlfeld (System) 1"=21900, "Auswählen"=1516, "Avogadro-Konstante (1/mol)"=23520, "Basis des natürlichen Logarithmus"=23510, "Basiseinheiten umwandeln"=1079, "Baumstruktur (Klassisch)"=21819, "Baumstruktur (Modern)"=21793, "Baumstruktur (System)"=21794, "Bedingte Deaktivierungsstruktur"=2064, "Benutzerdef. Referenz"=3428, "Benutzerdef. Referenz-Tag (Blockdiagrammkonstante)"=3426, "Benutzerdef. Referenz-Tag (Klassisch)"=3429, "Benutzerdef. Referenz-Tag (Modern)"=21745, "Benutzerdef. Tag (Blockdiagrammkonstante)"=2114, "Benutzerdef. Tag (Klassisch)"=3329, "Benutzerdef. Tag (Modern)"=21749, "Benutzerdefiniertes Trace-Ereignis erzeugen"=2250, "Benutzerereignis erstellen"=2073, "Benutzerereignis erzeugen"=2074, "Benutzerereignis löschen"=2075, "Benutzerobjekt"=3506, "Berechtigungen ermitteln"=8065, "Berechtigungen festlegen"=8076, "Bereich"=2196, "Bereich sperren"=1411, "Beschriftete Schaltfläche (Rechteck)"=3123, "Beschriftete Schaltfläche (Rund)"=3122, "Beschriftete Schaltfläche (runde Ecken)"=3124, "Beschriftete Schaltfläche (runde Kanten)"=3125, "Beschriftung (Modern)"=21960, "Beschriftung (System)"=21961, "Bildlaufleiste (horizontal)"=21110, "Bildlaufleiste (vertikal)"=21111, "Bis zum nächsten Vielfachen von ms warten"=1327, "Bitpack nach Array"=3135, "Bluetooth - Auf Listener warten"=9147, "Bluetooth - Erkennung"=9152, "Bluetooth - Lesen"=9149, "Bluetooth - Listener erstellen"=9151, "Bluetooth - Netzwerkverbindung (Referenz)"=3468, "Bluetooth - Schreiben"=9150, "Bluetooth - Verbindung beenden"=9148, "Bluetooth - Verbindung herstellen"=9153, "Boolescher Wert nach (0,1)"=1167, "Boolesches Array nach Zahl"=1815, "Bruch-/Exponential-String nach Zahl"=1187, "Byte-Array nach String"=1609, "Bytes tauschen"=1162, "Bytestream-Datei (Referenz)"=3408, "Bündeln"=2049, "CAN-Kanal (Blockdiagrammkonstante)"=2124, "CAN-Kanal (Klassisch)"=3340, "CAN-Kanal (Modern)"=21817, "CAN-Kanal (System)"=21966, "CAN-Schnittstelle (Blockdiagrammkonstante)"=2123, "CAN-Schnittstelle (Klassisch)"=3339, "CAN-Schnittstelle (Modern)"=21815, "CAN-Schnittstelle (System)"=21964, "CAN-Task (Blockdiagrammkonstante)"=3471, "CAN-Task (Klassisch)"=3470, "CAN-Task (Modern)"=21789, "CAN-Task (System)"=21963, "Case-Struktur"=2001, "Cluster (Klassisch)"=3400, "Cluster (Modern)"=21607, "Cluster nach Array"=1169, "Cluster-Array erstellen"=2047, "Cluster-Array indizieren und bündeln"=2056, "Cluster-Konstante"=2071, "Code-Interface-Knoten"=2050, "Cosecans"=1204, "Cosecans Hyperbolicus"=23053, "Cosinus"=1201, "Cosinus Hyperbolicus"=1215, "Cotangens"=1205, "Cotangens Hyperbolicus"=23055, "CPU-Informationen"=24130, "DAQ-Kanal (Traditionell) (Blockdiagrammkonstante)"=2085, "DAQ-Kanal (Traditionell) (Klassisch)"=3320, "DAQ-Kanal (Traditionell) (Modern)"=21733, "DAQmx - Analog-Trigger-Quelle (Blockdiagrammkonstante)"=2119, "DAQmx - Analog-Trigger-Quelle (Klassisch)"=3336, "DAQmx - Analog-Trigger-Quelle (Modern)"=21774, "DAQmx - Analog-Trigger-Quelle (System)"=21951, "DAQmx - Globaler Kanal (Blockdiagrammkonstante)"=3430, "DAQmx - Globaler Kanal (Klassisch)"=3443, "DAQmx - Globaler Kanal (Modern)"=21770, "DAQmx - Globaler Kanal (System)"=21957, "DAQmx - Physikalischer Kanal (Blockdiagrammkonstante)"=2118, "DAQmx - Physikalischer Kanal (Klassisch)"=3335, "DAQmx - Physikalischer Kanal (Modern)"=21777, "DAQmx - Physikalischer Kanal (System)"=21954, "DAQmx-Anschluss (Blockdiagrammkonstante)"=2117, "DAQmx-Anschluss (Klassisch)"=3319, "DAQmx-Anschluss (Modern)"=21781, "DAQmx-Anschluss (System)"=21955, "DAQmx-Gerätename (Blockdiagrammkonstante)"=2093, "DAQmx-Gerätename (Klassisch)"=3318, "DAQmx-Gerätename (Modern)"=21773, "DAQmx-Gerätename (System)"=21950, "DAQmx-Skalierungsname (Blockdiagrammkonstante)"=2116, "DAQmx-Skalierungsname (Klassisch)"=3317, "DAQmx-Skalierungsname (Modern)"=21775, "DAQmx-Skalierungsname (System)"=21952, "DAQmx-Switch (Blockdiagrammkonstante)"=2121, "DAQmx-Switch (Klassisch)"=3337, "DAQmx-Switch (Modern)"=21776, "DAQmx-Switch (System)"=21953, "DAQmx-Task-Name (Blockdiagrammkonstante)"=3434, "DAQmx-Task-Name (Klassisch)"=3442, "DAQmx-Task-Name (Modern)"=21778, "DAQmx-Task-Name (System)"=21959, "DataSocket-Referenz"=3417, "DataSocket: Lesen"=1086, "DataSocket: Schließen"=1085, "DataSocket: Schreiben"=1087, "DataSocket: Öffnen"=1084, "Datei lesen"=1407, "Datei schließen"=8052, "Datei schließen (veraltet)"=1405, "Datei schreiben"=1408, "Datei öffnen"=1403, "Datei- und Programmtyp"=1434, "Datei- und Programmtyp ermitteln"=8066, "Datei- und Programmtyp festlegen"=8077, "Datei-/Verzeichnis-Info"=8082, "Datei-/Verzeichnis-Info (veraltet)"=1413, "Dateidialog"=8058, "Dateidialog (veraltet)"=8081, "Dateigröße ermitteln"=8063, "Dateigröße festlegen"=8074, "Dateipfad-Anzeigeelement (Klassisch)"=3204, "Dateipfad-Anzeigeelement (Modern)"=21731, "Dateipfad-Bedienelement (Klassisch)"=3203, "Dateipfad-Bedienelement (Modern)"=21730, "Dateipfad-Bedienelement (System)"=21922, "Dateiposition ermitteln"=8062, "Dateiposition festlegen"=8073, "Dateipuffer leeren"=8059, "Dateipuffer leeren (veraltet)"=1406, "Daten serialisieren"=1164, "Daten-Cache-Größe"=24132, "Datenprotokoll lesen"=8069, "Datenprotokoll schreiben"=8079, "Datenprotokolldatei (Referenz)"=3402, "Datenträger-Info"=1414, "Datenträger-Info lesen"=8067, "Datenwertreferenz löschen"=2409, "Datum-/Zeit-String lesen"=1600, "Datum/Zeit formatieren"=8100, "Datum/Zeit in Sekunden ermitteln"=1303, "Datum/Zeit nach Sekunden"=1308, "Dekrementieren"=1058, "DevClear"=1961, "DevClearList"=1962, "Dezimal-String nach Zahl"=1184, "Dezimalzeichen gleich?"=23064, "Dezimalziffer?"=1119, "Diagrammdeaktivierungsstruktur"=2054, "Dialogfeld mit einer Schaltfläche"=1340, "Dialogfeld mit zwei Schaltflächen"=1341, "Digitaldaten (Klassisch)"=3210, "Digitaldaten (Modern)"=21216, "Digitaler Signalverlaufsgraph (Klassisch)"=3511, "Digitaler Signalverlaufsgraph (Modern)"=21718, "Dividieren"=1053, "Dividieren (mit Fehleranschlüssen)"=3918, "Dlg Horiz. Bildlaufleiste"=21905, "Dlg Numerisch 1"=2100, "Dlg Numerisch 2"=3006, "Dlg String"=2110, "Dlg Vert. Bildlaufleiste"=21906, "Drehknopf (Klassisch)"=3005, "Drehknopf (Modern)"=21000, "Drehregler (Klassisch)"=3050, "Drehregler (Modern)"=21732, "Drehspulinstrument (Klassisch)"=3030, "Drehspulinstrument (Modern)"=21008, "Dreieck (abwärts)"=3623, "Dreieck (aufwärts)"=3622, "Dreieck (links)"=3620, "Dreieck (rechts)"=3621, "Dreiecksrelief (abwärts)"=3615, "Dreiecksrelief (aufwärts)"=3614, "Dreiecksrelief (links)"=3612, "Dreiecksrelief (rechts)"=3613, "Druckbar?"=1124, "Druckschalter"=21001, "Druckschalter (rechteckig)"=3119, "Druckschalter (rechteckig) (Profil)"=3113, "Druckschalter (rund)"=3118, "Druckschalter (rund) (Profil)"=3112, "Drucktank (flach)"=3075, "Drucktank (Klassisch)"=3070, "Drucktank (Modern)"=21751, "Drucktank (schattiert)"=21753, "Dynamische FPGA-Schnittstellen-Umwandlung"=5690, "Eigenschaftsknoten"=1920, "Ein Element aus Stream auslesen"=23797, "Ein Element in Stream schreiben"=23798, "Einfacher horiz. Schieber"=3003, "Einfacher String"=2115, "Einfacher vert. Schieber"=3002, "Einfaches numerisches Feld"=2900, "Einheit umrechnen"=2059, "Element am Anfang einfügen"=9129, "Element aus Queue entfernen"=9113, "Element einfügen"=9111, "Element einfügen (verlustbehaftet)"=9130, "Elementarladung (C)"=23517, "Elementreferenz"=3419, "Elternmethode aufrufen"=2354, "Empfangen"=1974, "Empfangsendpunkt für Netzwerk-Stream erstellen"=23811, "EnableLocal"=1963, "EnableRemote"=1964, "Enum (Klassisch)"=3023, "Enum (Modern)"=21605, "Enum (System)"=3062, "Enum-Konstante"=2090, "EOF"=1410, "Ereignis-Callback (Referenz)"=3435, "Ereignis-Callback registrieren"=2078, "Ereignisdatenknoten"=2102, "Ereignisregistrierung aufheben"=2076, "Ereignisstruktur"=2052, "Ersten String suchen"=1532, "Erster Aufruf?"=1083, "Exklusiv-NICHT-ODER"=1073, "Exklusiv-ODER"=1063, "Exponential"=1211, "Exponential (Arg) -1"=1222, "FALSE-Konstante"=2006, "Farbfeld"=3013, "Farbfeld mit dünnem Rahmen"=2905, "Farbfeld mit Rahmen (Klassisch)"=3008, "Farbfeld mit Rahmen (Modern)"=21019, "Farbfeldkonstante"=2120, "Farbiges Rechteck (Fehler?)"=3625, "Farbrampe"=3022, "Fehler zusammenfassen"=2147, "Fehler-Ringkonstante"=2039, "Festkomma in Integer umwandeln"=5566, "Festkomma-Überlaufzustand einschließen"=5564, "Festkomma-Überlaufzustand entfernen"=5563, "Festkomma-Überlaufzustand löschen"=5562, "Festkommakomponenten erfassen"=11163, "Festkommaüberlauf?"=5565, "FieldPoint-I/O-Kanal (Blockdiagrammkonstante)"=3440, "FieldPoint-I/O-Kanal (Klassisch)"=3439, "FieldPoint-I/O-Kanal (Modern)"=21784, "FIFO (Referenz)"=3474, "FindLstn"=1965, "FindRQS"=1966, "Flache Sequenzstruktur"=2069, "Fließkantenrelief (horizontal)"=3633, "Fließkantenrelief (vertikal)"=3634, "For-Schleife"=2002, "Formelknoten"=2004, "FPGA-Referenz nach Session"=2322, "Freie Beschriftung"=2321, "Frontpanel-Aktivität generieren"=1329, "Förderband"=3827, "Für Ereignisse registrieren"=2065, "Gabelung"=2194, "Gerät lesen"=1432, "Gerät schreiben"=1431, "Gerät öffnen"=1430, "Gerätereferenz"=3405, "Gerätsteuerung/Status"=1433, "Gestapelte Sequenzstruktur"=2000, "Gleich 0?"=1113, "Gleich?"=1102, "Globale Variable"=2060, "GPIB: Initialisierung"=1957, "GPIB: Lesen"=1951, "GPIB: Schreiben"=1950, "GPIB: Serielles Pollen"=1955, "GPIB: Status"=1959, "GPIB: Trigger"=1953, "GPIB: Verschiedenes"=1956, "GPIB: Warten"=1958, "GPIB: Zurücksetzen"=1954, "Grafikring (Klassisch)"=3015, "Grafikring (Modern)"=21602, "Grafikring (System)"=21925, "Gravitationskonstante (N m2/kg2)"=23519, "Größen-Handle"=1603, "Größer als 0?"=1117, "Größer oder gleich 0?"=1114, "Größer oder gleich?"=1103, "Größer?"=1110, "Heizkessel"=3829, "Hexadezimal-String nach Zahl"=1185, "Hexadezimalziffer?"=1123, "Hilfefenster steuern"=1353, "Hinzufügen (mit Fehleranschlüssen)"=3915, "Horiz. Linie"=3821, "Horiz. Rohrleitung (flach)"=3810, "Horiz. Rohrleitung (schattiert)"=3710, "Horiz. Rundbox"=3636, "Horizontaler Trennbalken (Klassisch)"=21863, "Horizontaler Trennbalken (System)"=21865, "ID des aktuellen Prozessors"=24131, "IMAQ-Session"=3415, "Immer kopieren"=2400, "Implikation"=1080, "In Array einfügen"=3911, "In Binärdatei schreiben"=8078, "In Datei formatieren"=2083, "In Datei suchen"=2082, "In Großbuchstaben"=1188, "In Kleinbuchstaben"=1189, "In OLE-Variant"=8002, "In String formatieren"=2081, "In String suchen"=2080, "In Textdatei schreiben"=8080, "In XML konvertieren"=8400, "Inkrementieren"=1057, "Inline-C-Knoten"=2104, "Inplace-Elementstruktur"=2360, "Integer in Festkomma umwandeln"=5567, "Intensitätsdiagramm (Klassisch)"=3509, "Intensitätsdiagramm (Modern)"=21719, "Intensitätsgraph (Klassisch)"=3510, "Intensitätsgraph (Modern)"=21720, "Intervall #1"=3073, "Intervall #2"=21755, "IP nach String"=1710, "IrDA-Netzwerkverbindung (Referenz)"=3450, "IrDA: Auf Listener warten"=9143, "IrDA: Geräte suchen"=9141, "IrDA: Lesen"=9145, "IrDA: Listener erzeugen"=9140, "IrDA: Schreiben"=9146, "IrDA: Verbindung herstellen"=9142, "IrDA: Verbindung schließen"=9144, "IVI Session löschen"=8103, "Kehrwert"=1059, "Kehrwert von e"=23511, "Kehrwert von Pi"=23507, "Kein Pfad (Konstante)"=23524, "Keine Referenz (Konstante)"=23526, "Keine Umgebungsvariable"=23527, "Keine Zahl/Kein Pfad/Keine Referenz?"=1128, "Kippschalter"=21002, "Kippschalter (vertikal)"=21740, "Klassenbezeichner-Konstante"=2094, "Kleiner als 0?"=1118, "Kleiner oder gleich 0?"=1115, "Kleiner oder gleich?"=1104, "Kleiner?"=1111, "Knoten zum Aufruf externer Bibliotheken"=2062, "Kombinationsfeld (Klassisch)"=3304, "Kombinationsfeld (Modern)"=21604, "Kombinationsfeld (System)"=21917, "Kombinationsfeldkonstante"=2088, "Komplex nach polar"=1045, "Komplex nach Re/Im"=1044, "Komplex-Konjugierte"=1048, "Kompressor"=3832, "Konstruktorknoten"=3904, "Kopieren"=8053, "Kopieren (veraltet)"=1416, "Kreis"=3605, "Kreisförmiges Relief"=3603, "Kreuzung"=2197, "LabVIEW beenden"=1352, "LabVIEW-Objekt"=3457, "Laufzeitklasse erhalten"=8018, "Leak Variant Value Reference"=2410, "LED (rechteckig) (Klassisch)"=3121, "LED (rechteckig) (Modern)"=21013, "LED (rund) (Klassisch)"=3120, "LED (rund) (Modern)"=21012, "LED-Schalter"=3116, "Leerer Pfad (Konstante)"=23523, "Leerer String (Konstante)"=23503, "Leerer String/Pfad?"=1112, "Leeres Array?"=23063, "Leuchte (rechteckig)"=3105, "Leuchte (rund)"=3104, "Lexikalische Klasse"=1126, "Lichtgeschwindigkeit im Vakuum (m/s)"=23518, "Linie (dick)"=3629, "Linie (dünn)"=3626, "Linie (vertieft) (System)"=3632, "Linie (vertieft, dick)"=3630, "Linie (vertieft, dünn)"=3627, "Linie mit Pfeil (dick)"=3631, "Linie mit Pfeil (dünn)"=3628, "Listenfeld (Klassisch)"=21806, "Listenfeld (Modern)"=21792, "Listenfeld (System)"=21805, "Listenfeldsymbol-Ringkonstante"=2038, "Logarithmus zur Basis 10"=1210, "Logarithmus zur Basis 10 von e"=23512, "Logarithmus zur Basis 2"=1225, "Logarithmus zur Basis x"=1224, "Logischer IVI-Name (Blockdiagrammkonstante)"=3420, "Logischer IVI-Name (Klassisch)"=3414, "Logischer IVI-Name (Modern)"=21736, "Logisches Verschieben"=1081, "Lokale Variable"=2061, "Löschen"=8056, "Löschen (veraltet)"=1417, "Mantisse und Exponent"=1150, "Maschinengenauigkeit"=23528, "MathScript-Aufruf über Referenzknoten"=3906, "MathScript-Knoten"=2357, "MATLAB-Skript"=9020, "Matrix entpacken"=23000, "Matrix erstellen"=8500, "Matrix transponieren"=8509, "Matrixdiagonale festlegen"=8504, "Matrixdiagonale lesen"=8501, "Matrixelemente festlegen"=8505, "Matrixelemente lesen"=8502, "Matrixgröße"=8507, "Matrixgröße ändern"=8508, "Max & Min"=1108, "Max. & Min. von Array"=1907, "Mehrere Elemente aus Stream auslesen"=23803, "Mehrere Elemente in Stream schreiben"=23804, "Mehrfacharithmetik"=2200, "Mehrsegmentrohr"=23780, "Mehrspaltiges Listenfeld (Klassisch)"=21799, "Mehrspaltiges Listenfeld (Modern)"=21791, "Mehrspaltiges Listenfeld (System)"=21798, "Melder anfordern"=9101, "Melder freigeben"=9102, "Melderreferenz"=3423, "Melderstatus lesen"=9103, "Meldung abbrechen"=9107, "Meldung senden"=9104, "Menü-Popup-Ring"=3017, "Menüauswahl abfragen"=9001, "Menüleiste des aktuellen VIs"=9000, "Menüpunkt-Info lesen"=9005, "Menüpunkte einfügen"=9003, "Menüpunkte löschen"=9004, "Menüpunkteinstellungen"=9006, "Menüreferenz"=3413, "Menüring (Klassisch)"=3018, "Menüring (Modern)"=21600, "Menüverknüpfung abfragen"=9007, "Messleiste (horizontal)"=21106, "Messleiste (vertikal)"=21107, "Methodenknoten"=3900, "Mischsignalgraph"=21721, "Mit Potenz von 2 multiplizieren"=1074, "Molare Gas-Konstante (J/(mol K))"=23522, "Motion-Ressource (Blockdiagrammkonstante)"=3449, "Motion-Ressource (Klassisch)"=3448, "Motion-Ressource (Modern)"=21787, "Motor (flach)"=3820, "Motor (schattiert)"=3720, "Multifrequenzstruktur"=2199, "Multiplizieren"=1052, "Multiplizieren (mit Fehleranschlüssen)"=3917, "Muster suchen"=1535, "Nach allgemeinerer Klasse"=8017, "Nach Byte-Integer"=1140, "Nach Festkomma"=5561, "Nach Fließkommawert (doppelte Genauigkeit)"=1147, "Nach Fließkommawert (einfache Genauigkeit)"=1146, "Nach Fließkommawert (erweitert)"=1149, "Nach Komplex (doppelte Genauigkeit)"=1152, "Nach Komplex (einfache Genauigkeit)"=1151, "Nach Komplex (höchste Genauigkeit)"=1154, "Nach links rotieren (mit Übertrag)"=1606, "Nach Long-Integer"=1142, "Nach Namen aufschlüsseln"=2058, "Nach Namen bündeln"=2057, "Nach Quad-Integer"=1155, "Nach rechts rotieren (mit Übertrag)"=1607, "Nach Sonden-String"=2413, "Nach spezifischerer Klasse"=8016, "Nach Variant"=8201, "Nach vorzeichenlosen Byte-Integer"=1143, "Nach vorzeichenlosen Long-Integer"=1145, "Nach vorzeichenlosen Quad-Integer"=1156, "Nach vorzeichenlosen Wort-Integer"=1144, "Nach Wert durchsuchen"=1534, "Nach Wort-Integer"=1141, "Nach Zeitstempel"=5560, "Natürlicher Logarithmus"=1209, "Natürlicher Logarithmus (Arg +1)"=1221, "Natürlicher Logarithmus von 10"=23513, "Natürlicher Logarithmus von 2"=23514, "Natürlicher Logarithmus von Pi"=23508, "Negativ unendlich"=23509, "Negieren"=1069, "Neue Datei"=1404, "Neue Datenwertreferenz"=2408, "Neue IVI-Session"=8102, "Neues Verzeichnis"=1402, "Neues VI"=8014, "Neues VI-Objekt"=8015, "NICHT"=1064, "Nicht darstellbares Zeichen?"=1125, "Nicht-ODER"=1072, "Nicht-UND"=1071, "Numerische Konstante"=2005, "Numerisches Anzeigeelement (Klassisch)"=3001, "Numerisches Anzeigeelement (Modern)"=21004, "Numerisches Bedienelement (Klassisch)"=3000, "Numerisches Bedienelement (Modern)"=21003, "Numerisches Bedienelement (System)"=21919, "Occurrence (Referenz)"=3406, "Occurrence erzeugen"=1700, "Occurrence festlegen"=1702, "ODER"=1062, "ODER (Array-Elemente)"=1910, "Offener Tank (flach) (Klassisch)"=21752, "Offener Tank (schattiert) (Klassisch)"=3074, "OK-Schaltfläche (Modern)"=21738, "OK-Schaltfläche (System)"=3130, "Oktal-String nach Zahl"=1186, "Oktalziffer?"=1129, "OLE-Variant"=3150, "Online-Hilfe steuern"=1355, "Optionsfeld (rechteckig)"=3107, "Optionsfeld (rund)"=3106, "Optionsfeld (System)"=3133, "Optionsfelder (Klassisch)"=22003, "Optionsfelder (Modern)"=22001, "Optionsfelder (System)"=22002, "Ordner anzeigen"=8083, "Ordner erstellen"=8055, "Paketmatrix"=23001, "PassControl"=1968, "Peek-Operation verarbeiten"=1604, "Pfad des aktuellen VIs"=1426, "Pfad erstellen"=1419, "Pfad nach Array aus Strings"=1423, "Pfad nach String"=1077, "Pfad zerlegen"=1420, "Pfadkonstante"=2009, "Pfadtyp"=1421, "Pfeil (Abwärts)"=3824, "Pfeil (aufwärts)"=3823, "Pfeil (links)"=3826, "Pfeil (rechts)"=3825, "Pi"=23504, "Pi geteilt durch 2"=23506, "Pi multipliziert mit 2"=23505, "PixMap"=3505, "PixMap (Warnung: gefährlich)"=3507, "Planck-Konstante (J/Hz)"=23516, "Plattform: Flache Rechteck-Schaltfläche"=3134, "Plugin-Steuerung"=21820, "Poke-Operation verarbeiten"=1605, "Polar nach komplex"=1047, "Polar nach Re/Im"=23061, "Position im Datenprotokoll ermitteln"=8061, "Position im Datenprotokoll festlegen"=8072, "Positiv unendlich"=23515, "Potenz von 10"=1212, "Potenz von 2"=1223, "PPoll"=1969, "PPollConfig"=1970, "PPollUnconfig"=1971, "Pulldown-Menüring"=3061, "Pumpe (links) (flach)"=3813, "Pumpe (links) (schattiert)"=3713, "Pumpe (rechts) (flach)"=3819, "Pumpe (rechts) (schattiert)"=3719, "Quadrat"=23059, "Quadratwurzel"=1060, "Queue anfordern"=9108, "Queue freigeben"=9109, "Queue leeren"=9114, "Queue-Referenz"=3424, "Queue-Status lesen"=9110, "Quotient und Rest"=1056, "Rahmen"=3608, "RcvRespMsg"=1972, "Re/Im nach komplex"=1046, "Re/Im nach polar"=23060, "ReadStatus"=1973, "ReceiveSetup"=1975, "Rechteck"=3602, "Rechteckschaltfläche"=3103, "Referenz nach Pfad"=1424, "Referenz nach Session"=2306, "Referenz schließen"=8011, "Regel- und Simulationsschleife"=2099, "Registerkartenelement (Klassisch)"=3330, "Registerkartenelement (Modern)"=3332, "Registerkartenelement (System)"=3331, "Registrierung für Sitzung entfernen"=2320, "Registrierungssession"=2319, "Reliefrahmen"=3606, "ResetSys"=1976, "Ressourcen-Index"=1088, "Rohrknie (links, abwärts) (flach)"=3811, "Rohrknie (links, abwärts) (schattiert)"=3711, "Rohrknie (links, aufwärts) (flach)"=3708, "Rohrknie (links, aufwärts) (flach) 1"=3808, "Rohrknie (rechts, abwärts) (flach)"=3817, "Rohrknie (rechts, abwärts) (schattiert)"=3717, "Rohrknie (rechts, aufwärts) (flach)"=3814, "Rohrknie (rechts, aufwärts) (schattiert)"=3714, "Rotationsverteiler"=3830, "Rotieren"=1082, "RT-FIFO erstellen"=24000, "RT-FIFO lesen"=24001, "RT-FIFO löschen"=24003, "RT-FIFO schreiben"=24002, "Rundinstrument (Klassisch)"=3040, "Rundinstrument (Modern)"=21009, "Rundschaltfläche"=3102, "Rydberg-Konstante (1/m)"=23521, "Rückkopplungsknoten"=2353, "Schalter (horizontal)"=3108, "Schalter (vertikal)"=3109, "Schaltfläche (rechteckig)"=3101, "Schaltfläche (rund)"=3100, "Schieber (horizontal) (Klassisch)"=3010, "Schieber (horizontal) (System)"=21904, "Schieber (horizontal, gefüllt) (Klassisch)"=3012, "Schieber (horizontal, gefüllt) (Modern)"=21100, "Schieber (vertikal) (System)"=21903, "Schieber (vertikal, gefüllt) (Klassisch)"=3009, "Schieber (vertikal, gefüllt) (Modern)"=21014, "Schieber mit Knopf (vertikal)"=3004, "Schieber mit Zeiger (horizontal) (Klassisch)"=3011, "Schieber mit Zeiger (horizontal) (Modern)"=21101, "Schieber mit Zeiger (horizontal) (System)"=21902, "Schieber mit Zeiger (vertikal) (Klassisch)"=3007, "Schieber mit Zeiger (vertikal) (Modern)"=21017, "Schieber mit Zeiger (vertikal) (System)"=21901, "Schiebeschalter"=21011, "Schiebeschalter (horizontal)"=3114, "Schiebeschalter (vertikal) (Klassisch)"=3115, "Schiebeschalter (vertikal) (Modern)"=21741, "Schwellwert (1D-Array)"=1909, "Secans"=1203, "Secans Hyperbolicus"=23054, "Sekunden nach Datum/Zeit"=1309, "SendCmds"=1978, "SendDataBytes"=1979, "Sendeendpunkt für Netzwerk-Stream erstellen"=23810, "Senden"=1977, "SendIFC"=1980, "SendList"=1981, "SendLLO"=1982, "SendSetup"=1983, "Serialisierte Daten nach Variant"=8202, "Serialisiertes benutzerdef. Referenz-Tag (Klassisch)"=3454, "Serialisiertes benutzerdef. Referenz-Tag (Modern)"=21747, "Session nach Referenz"=2307, "SetRWLS"=1984, "SetTimeOut"=1985, "Signale trennen"=2351, "Signale zusammenfassen"=2350, "Signalverlauf erstellen"=2066, "Signalverlaufsattribut entfernen"=8209, "Signalverlaufsattribut ermitteln"=8208, "Signalverlaufsattribut festlegen"=8207, "Signalverlaufsdiagramm"=21010, "Signalverlaufsdiagramm (Klassisch)"=3501, "Signalverlaufsdiagramm (Modern)"=21717, "Signalverlaufsgraph (Klassisch)"=3504, "Signalverlaufsgraph (Modern)"=21703, "Signalverlaufskomponenten lesen"=2067, "Sinc"=1227, "Sinus"=1200, "Sinus Hyperbolicus"=1214, "Sinus und Cosinus"=1220, "Speicherfreigabe anfordern"=1610, "Standardverzeichnis"=1427, "Statische VI-Referenz"=2084, "Status des Hilfefensters lesen"=1354, "Stopp"=1350, "Stopp-Schaltfläche"=21230, "Stopp-Schaltfläche (rechteckig)"=3128, "Stopp-Schaltfläche (rund)"=3127, "Stream beenden"=23807, "Stream erstellen"=23796, "Stream leeren"=23808, "Stream prüfen und verknüpfen"=23805, "Stream starten"=23806, "Stream verknüpfen"=23793, "Stream-Endpunkt entfernen"=23794, "Stream-Verknüpfung aufheben"=23795, "String deserialisieren"=1165, "String durchsuchen und teilen"=1538, "String nach Byte-Array"=1608, "String nach IP"=1711, "String nach Pfad"=1078, "String nach Token durchsuchen"=8101, "String nach Umgebungsvariable"=1830, "String rotieren"=1536, "String suchen und ersetzen"=3914, "String umkehren"=1537, "String-Anzeigeelement (Klassisch)"=3201, "String-Anzeigeelement (Modern)"=21702, "String-Array indizieren"=1531, "String-Bedienelement (Klassisch)"=3200, "String-Bedienelement (Modern)"=21701, "String-Bedienelement (System)"=21920, "String-Konstante"=2007, "String-Länge"=1502, "Stringarray sortieren"=23065, "Strings verknüpfen"=2040, "Subtrahieren"=1051, "Subtrahieren (mit Fehleranschlüssen)"=3916, "Suchen"=1409, "T-Stück (abwärts) (flach)"=3818, "T-Stück (abwärts) (schattiert)"=3718, "T-Stück (aufwärts) (flach)"=3812, "T-Stück (aufwärts) (schattiert)"=3712, "T-Stück (links) (flach)"=3809, "T-Stück (links) (schattiert)"=3709, "T-Stück (rechts) (flach)"=3815, "T-Stück (rechts) (schattiert)"=3715, "Tabelle (Klassisch)"=21796, "Tabelle (Modern)"=21790, "Tabelle (System)"=21797, "Tabellen-String nach Array"=1539, "Tabulatorkonstante"=23502, "Tag-Attributring"=2063, "Tangens"=1202, "Tangens Hyperbolicus"=1216, "Tank (horizontal)"=3071, "Tank (Klassisch)"=3020, "Tank (Modern)"=21006, "TCP-Netzwerkverbindung (Referenz)"=3407, "TCP: Auf Listener warten"=1712, "TCP: Lesen"=1716, "TCP: Lesen (Flex.)"=1720, "TCP: Lesen (Strings)"=1718, "TCP: Listener erstellen"=1717, "TCP: Schreiben"=1714, "TCP: Schreiben (Flex.)"=1721, "TCP: Schreiben (Strings)"=1719, "TCP: Verbindung herstellen"=1715, "TCP: Verbindung schließen"=1713, "TDMS Close"=24113, "TDMS Defragment"=24119, "TDMS Flush"=24117, "TDMS Get Properties"=24115, "TDMS List Contents"=24116, "TDMS Open"=24112, "TDMS Read"=24111, "TDMS Refnum To File ID"=24120, "TDMS Set Properties"=24114, "TDMS Write"=24110, "TDMS Write IP"=24118, "TDMS: Datei"=3477, "Teil-Array"=2044, "Teil-Array ersetzen"=3910, "Teil-String"=1503, "Teil-String ersetzen"=3913, "Temporäres Verzeichnis"=1435, "TestSRQ"=1986, "TestSys"=1987, "Text nach UTF-8"=23066, "Text- & Grafikring (Klassisch)"=3016, "Text- & Grafikring (Modern)"=21603, "Text-Schaltfläche"=21015, "Textring (Blockdiagrammkonstante)"=2008, "Textring (Klassisch)"=3014, "Textring (Modern)"=21601, "Textring (System)"=3060, "Thermometer (Klassisch)"=3021, "Thermometer (Modern)"=21007, "Timer-Wert (ms)"=1300, "Trennbalken (horizontal)"=21861, "Trennbalken (vertikal)"=21860, "Trennschalter"=21020, "Trichter 1"=21754, "Trichter 2"=3072, "Trigger"=1988, "TriggerList"=1989, "TRUE/FALSE-String anhängen"=1511, "TRUE/FALSE-String suchen"=1533, "Typ erzwingen"=2402, "Typumwandlung"=1166, "UDP-Netzwerkverbindung (Referenz)"=3418, "UDP: Lesen"=1724, "UDP: Multicast öffnen"=1727, "UDP: Schließen"=1726, "UDP: Schreiben"=1725, "UDP: Öffnen"=1723, "Umgebungsvariable"=23778, "Umgebungsvariable nach String"=1831, "Umgebungsvariablenelement (Klassisch)"=3472, "Umgebungsvariablenelement (Modern)"=21814, "Umgebungsvariablenkonstante"=3473, "Umschalter (horizontal) (Klassisch)"=3110, "Umschalter (horizontal) (Modern)"=21700, "Umschalter (vertikal) (Klassisch)"=3111, "Umschalter (vertikal) (Modern)"=21005, "Unbitpack von Array"=3136, "UND"=1061, "UND (Array-Elemente)"=1911, "Ungleich 0?"=1116, "Ungleich?"=1105, "Unleak Variant Value Reference"=2411, "Untermatrix festlegen"=8506, "Untermatrix lesen"=8503, "Unterpanel"=21810, "Unterpanel (klassisch)"=21811, "Unterpanel (System)"=21823, "UTF-8 nach Text"=23067, "Variable auslesen (mit Timeout)"=23786, "Variable direkt lesen"=23785, "Variable direkt schreiben"=23788, "Variable lesen"=23781, "Variable lesen (Scan)"=23784, "Variable schreiben"=23782, "Variable schreiben (mit Timeout)"=23789, "Variable schreiben (Scan)"=23787, "Variablen-Container suchen"=23802, "Variablenklassenbezeichner-Konstante"=2106, "Variablenkonfiguration"=3475, "Variablenname (Konstante)"=3478, "Variablenverbindung beenden"=23783, "Variablenverbindung herstellen"=23779, "Variablenverbindung herstellen und prüfen"=23790, "Variablenverbindung im Hintergrund herstellen"=23791, "Variant"=3310, "Variant nach Daten"=8003, "Variant nach serialisierte Daten"=8203, "Variant wieder zusammensetzen (Warnung: gefährlich)"=2405, "Variant zerlegen"=2404, "Variantattribut entfernen"=8206, "Variantattribut ermitteln"=8205, "Variantattribut festlegen"=8204, "Vektorwerte austauschen"=1912, "Ventil (Abwärtsbogen) (flach)"=3707, "Ventil (Abwärtsbogen) (schattiert)"=21767, "Ventil (Abwärtsbogen) (Umriss)"=3807, "Ventil (Aufwärtsbogen) (flach)"=3703, "Ventil (Aufwärtsbogen) (schattiert)"=21763, "Ventil (Aufwärtsbogen) (Umriss)"=3803, "Ventil (Linksbogen) (flach)"=3701, "Ventil (Linksbogen) (schattiert)"=21761, "Ventil (Linksbogen) (Umriss)"=3801, "Ventil (Rechtsbogen) (flach)"=3705, "Ventil (Rechtsbogen) (schattiert)"=21765, "Ventil (Rechtsbogen) (Umriss)"=3805, "Ventil (rechtwinklig, abwärts) (flach)"=3706, "Ventil (rechtwinklig, abwärts) (schattiert)"=21766, "Ventil (rechtwinklig, abwärts) (Umriss)"=3806, "Ventil (rechtwinklig, aufwärts) (flach)"=3702, "Ventil (rechtwinklig, aufwärts) (schattiert)"=3802, "Ventil (rechtwinklig, aufwärts) (Umriss)"=21762, "Ventil (rechtwinklig, links) (flach)"=3700, "Ventil (rechtwinklig, links) (schattiert)"=21760, "Ventil (rechtwinklig, links) (Umriss)"=3800, "Ventil (rechtwinklig, rechts) (flach)"=3704, "Ventil (rechtwinklig, rechts) (schattiert)"=21764, "Ventil (rechtwinklig, rechts) (Umriss)"=3804, "Ventil prüfen"=3833, "Vereinigung"=2195, "Verlaufsanzeige (horizontal) (Modern)"=21102, "Verlaufsanzeige (horizontal) (System)"=21910, "Verlaufsanzeige (vertikal) (Modern)"=21104, "Verlaufsanzeige (vertikal) (System)"=21909, "Verschieben"=8068, "Verschieben (veraltet)"=1415, "Verschobene Daten ermitteln"=9154, "Vert. Linie"=3822, "Vert. Rohrleitung (flach)"=3816, "Vert. Rohrleitung (schattiert)"=3716, "Vertikaler Trennbalken (Klassisch)"=21862, "Vertikaler Trennbalken (System)"=21864, "Verzeichnis auflisten"=1418, "VI-Bibliothek"=1425, "VI-Objektreferenz öffnen"=8013, "VI-Referenz"=3422, "VI-Referenz öffnen"=8010, "VI-Server-Referenz"=2091, "Viereckiges Relief (Klassisch)"=3600, "Viereckiges Relief (Modern)"=3637, "Viereckiges Relief (runde Ecken)"=3609, "VISA-Referenz nach Session"=2300, "VISA-Ressourcenname"=3421, "VISA-Ressourcenname (Klassisch)"=3409, "VISA-Ressourcenname (Modern)"=21737, "VISA: Adresse freigeben"=1933, "VISA: Adresse zuweisen"=1932, "VISA: Auf Ereignis warten"=1943, "VISA: Bereich lesen (16)"=1948, "VISA: Bereich lesen (32)"=1991, "VISA: Bereich lesen (64)"=2144, "VISA: Bereich lesen (8)"=1946, "VISA: Bereich schreiben (16)"=1949, "VISA: Bereich schreiben (32)"=1992, "VISA: Bereich schreiben (64)"=2145, "VISA: Bereich schreiben (8)"=1947, "VISA: Ereignis aktivieren"=1942, "VISA: Ereignis deaktivieren"=1940, "VISA: Ereignis verwerfen"=1941, "VISA: GPIB sendet IFC"=2318, "VISA: GPIB steuert ATN"=2316, "VISA: GPIB steuert REN"=2304, "VISA: GPIB-Befehl"=2315, "VISA: GPIB-Durchgangssteuerung"=2317, "VISA: Hilfssignal anfordern"=2310, "VISA: I/O-Puffer entleeren"=2302, "VISA: I/O-Puffergröße festlegen"=2301, "VISA: In Datei lesen"=2313, "VISA: Interrupt anfordern"=2309, "VISA: Lesen"=1925, "VISA: Peek (16)"=1934, "VISA: Peek (32)"=1995, "VISA: Peek (64)"=2142, "VISA: Peek (8)"=1938, "VISA: Poke (16)"=1935, "VISA: Poke (32)"=1996, "VISA: Poke (64)"=2143, "VISA: Poke (8)"=1939, "VISA: Ressource suchen"=1923, "VISA: Schließen"=1922, "VISA: Schreiben"=1926, "VISA: Speicher freigeben"=1998, "VISA: Speicher reservieren"=1997, "VISA: Speicher reservieren (Ex)"=2146, "VISA: Sperre aufheben"=1994, "VISA: Sperren"=1993, "VISA: Statusinformation"=1924, "VISA: STB lesen"=1928, "VISA: Trigger freigeben"=2312, "VISA: Trigger freigeben 1"=1929, "VISA: Trigger zuweisen"=2311, "VISA: USB-Steuerung (Ausgang)"=2087, "VISA: USB-Steuerung (Eingang)"=2086, "VISA: Verschieben"=2303, "VISA: Von Datei schreiben"=2314, "VISA: VXI-Befehl oder -Abfrage"=2305, "VISA: Wert lesen (16)"=1930, "VISA: Wert lesen (32)"=1944, "VISA: Wert lesen (64)"=2140, "VISA: Wert lesen (8)"=1936, "VISA: Wert schreiben (16)"=1931, "VISA: Wert schreiben (32)"=1945, "VISA: Wert schreiben (64)"=2141, "VISA: Wert schreiben (8)"=1937, "VISA: Zurücksetzen"=1927, "VISA: Öffnen"=2308, "VISA: Öffnen (alt)"=1921, "Vorschau für Queue-Element"=9112, "Vorzeichen"=1049, "Wagenrücklauf-Konstante"=23500, "WaitSRQ"=1990, "Warten (ms)"=1302, "Wert formatieren"=1512, "Werte austauschen"=2401, "Wertebereich prüfen und erzwingen"=1127, "While-Schleife 1"=2003, "While-Schleife 2"=2352, "Words tauschen"=1163, "X hoch Y"=1213, "XY-Graph (Klassisch)"=3500, "XY-Graph (Modern)"=21716, "Y-te Wurzel von X"=23062, "Zahl nach boolesches Array"=1814, "Zahl nach Hexadezimal-String"=1181, "Zahl nach Oktal-String"=1182, "Zahl nach String (Dezimaldarstellung)"=1180, "Zahl nach String (Exponentialdarstellung)"=1505, "Zahl nach String (Fließkommadarstellung)"=1506, "Zahl nach String (Technische Notation)"=1183, "Zahl teilen"=1170, "Zahlen verbinden"=1171, "Zeile auswählen"=1510, "Zeilenende-Konstante"=23525, "Zeilenvorschub-Konstante"=23501, "Zeitgesteuerte Schleife"=5570, "Zeitgesteuerte Sequenz"=5573, "Zeitstempel (Blockdiagrammkonstante)"=2068, "Zeitstempel-Anzeigeelement (Klassisch)"=5556, "Zeitstempel-Anzeigeelement (Modern)"=21914, "Zeitstempel-Bedienelement (Klassisch)"=5555, "Zeitstempel-Bedienelement (modern)"=21913, "Zeitstempel-Bedienelement (System)"=21967, "ZerlegenGesperrteDatenWertRef"=2406, "Zufallszahl (0-1)"=1070, "Zugriff verweigern"=8057, "Zugriffsrechte"=1412, "ZusammensetzenSperreAufhebenDatenWertRef (Warnung: gefährlich)"=2407, "Zustand"=2198, "Zustandsdiagramm"=2051, "Öffnen/Erstellen/Ersetzen einer Datei"=8050, "Öffnen/Erstellen/Ersetzen einer Protokolldatei"=8054]
        w70 = refnum<vi> refnum  # NumericConstant
        w65 = 2005 items=[".NET (Referenz)"=3441, ".NET-Container"=2125, "1D-Array dezimieren"=2046, "1D-Array durchsuchen"=1901, "1D-Array interpolieren"=1905, "1D-Array rotieren"=1906, "1D-Array sortieren"=1120, "1D-Array teilen"=1908, "1D-Array transponieren"=23068, "1D-Array umkehren"=1900, "1D-Arrays überführen"=2045, "2D-Array transponieren"=1902, "2D-Bild"=3508, "3-Zustands-Feld (System)"=21333, "3D-Bild"=23776, "Abbrechen-Schaltfläche (Modern)"=21739, "Abbrechen-Schaltfläche (System)"=3131, "Abgerundetes Rechteck"=3611, "Abgesenkter Kreis"=3604, "Abgesenkter Menüring"=3019, "Abgesenkter Rahmen (Modern)"=3607, "Abgesenkter Rahmen (System)"=3624, "Abgesenktes abgerundetes Rechteck"=3638, "Abgesenktes Dreieck (abwärts)"=3619, "Abgesenktes Dreieck (aufwärts)"=3618, "Abgesenktes Dreieck (links)"=3616, "Abgesenktes Dreieck (rechts)"=3617, "Abgesenktes Rechteck (dick)"=3635, "Abgesenktes Viereck"=3601, "Abgesenktes Viereck (abgerundet)"=3610, "Absoluter Wert"=1054, "ActiveX (Referenz)"=3410, "ActiveX-Container"=2072, "ActiveX-Objekt schließen"=8001, "ActiveX-Objekt öffnen"=8000, "Addieren"=1050, "AdrErstellen"=1967, "Agitator"=3831, "Aktivieren der Menüüberwachung"=9002, "AllSpoll"=1960, "Anzahl der Cache-Level"=24133, "Anzahl der Datensätze ermitteln"=8064, "Anzahl der Datensätze festlegen"=8075, "Applikationsreferenz"=3412, "Applikationsreferenz öffnen"=8012, "Arcuscosecans"=23050, "Arcuscosinus"=1207, "Arcuscotangens"=23052, "Arcussecans"=23051, "Arcussinus"=1206, "Arcustangens"=1208, "Arcustangens (2 Eingänge)"=1228, "Areacosecans"=23056, "Areacosinus Hyperbolicus"=1218, "Areacotangens"=23058, "Areasecans"=23057, "Areasinus Hyperbolicus"=1217, "Areatangens Hyperbolicus"=1219, "Array (Blockdiagrammkonstante)"=2070, "Array (Klassisch)"=3300, "Array (Modern)"=21608, "Array aus Strings nach Pfad"=1422, "Array erstellen"=2041, "Array indizieren"=2042, "Array initialisieren"=2053, "Array Interface Control"=23777, "Array nach Cluster"=1168, "Array nach Tabellen-String"=1540, "Array umformen"=2055, "Array wieder zusammensetzen"=2403, "Array zerlegen"=2412, "Array-Elemente addieren"=1903, "Array-Elemente multiplizieren"=1904, "Array-Größe"=1809, "Auf Aktion warten"=1722, "Auf Frontpanel-Aktivität warten"=1328, "Auf GPIB-RQS warten"=1952, "Auf Meldung mit Melderhistorie warten"=9131, "Auf Meldung von mehreren mit Melderhistorie warten"=9132, "Auf Meldung von mehreren warten"=9106, "Auf Meldung warten"=9105, "Auf nächste ganze Zahl runden"=1055, "Auf nächstgrößere Zahl runden"=1076, "Auf nächstkleinere Zahl runden"=1075, "Auf Occurrence warten"=1701, "Auf Stream-Status warten"=23809, "Auf Stream-Verknüpfung warten"=23799, "Aufruf über Referenz"=3901, "Aufrufkette"=1999, "Aufschlüsseln"=2048, "Aus Array entfernen"=3912, "Aus Binärdatei lesen"=8051, "Aus Textdatei lesen"=8070, "Aus XML zurückkonvertieren"=8401, "Ausdrucksknoten"=2201, "Austauscher"=3828, "Auswahlfeld (Klassisch)"=3117, "Auswahlfeld (Modern)"=21924, "Auswahlfeld (System)"=3132, "Auswahlfeld (System) 1"=21900, "Auswählen"=1516, "Avogadro-Konstante (1/mol)"=23520, "Basis des natürlichen Logarithmus"=23510, "Basiseinheiten umwandeln"=1079, "Baumstruktur (Klassisch)"=21819, "Baumstruktur (Modern)"=21793, "Baumstruktur (System)"=21794, "Bedingte Deaktivierungsstruktur"=2064, "Benutzerdef. Referenz"=3428, "Benutzerdef. Referenz-Tag (Blockdiagrammkonstante)"=3426, "Benutzerdef. Referenz-Tag (Klassisch)"=3429, "Benutzerdef. Referenz-Tag (Modern)"=21745, "Benutzerdef. Tag (Blockdiagrammkonstante)"=2114, "Benutzerdef. Tag (Klassisch)"=3329, "Benutzerdef. Tag (Modern)"=21749, "Benutzerdefiniertes Trace-Ereignis erzeugen"=2250, "Benutzerereignis erstellen"=2073, "Benutzerereignis erzeugen"=2074, "Benutzerereignis löschen"=2075, "Benutzerobjekt"=3506, "Berechtigungen ermitteln"=8065, "Berechtigungen festlegen"=8076, "Bereich"=2196, "Bereich sperren"=1411, "Beschriftete Schaltfläche (Rechteck)"=3123, "Beschriftete Schaltfläche (Rund)"=3122, "Beschriftete Schaltfläche (runde Ecken)"=3124, "Beschriftete Schaltfläche (runde Kanten)"=3125, "Beschriftung (Modern)"=21960, "Beschriftung (System)"=21961, "Bildlaufleiste (horizontal)"=21110, "Bildlaufleiste (vertikal)"=21111, "Bis zum nächsten Vielfachen von ms warten"=1327, "Bitpack nach Array"=3135, "Bluetooth - Auf Listener warten"=9147, "Bluetooth - Erkennung"=9152, "Bluetooth - Lesen"=9149, "Bluetooth - Listener erstellen"=9151, "Bluetooth - Netzwerkverbindung (Referenz)"=3468, "Bluetooth - Schreiben"=9150, "Bluetooth - Verbindung beenden"=9148, "Bluetooth - Verbindung herstellen"=9153, "Boolescher Wert nach (0,1)"=1167, "Boolesches Array nach Zahl"=1815, "Bruch-/Exponential-String nach Zahl"=1187, "Byte-Array nach String"=1609, "Bytes tauschen"=1162, "Bytestream-Datei (Referenz)"=3408, "Bündeln"=2049, "CAN-Kanal (Blockdiagrammkonstante)"=2124, "CAN-Kanal (Klassisch)"=3340, "CAN-Kanal (Modern)"=21817, "CAN-Kanal (System)"=21966, "CAN-Schnittstelle (Blockdiagrammkonstante)"=2123, "CAN-Schnittstelle (Klassisch)"=3339, "CAN-Schnittstelle (Modern)"=21815, "CAN-Schnittstelle (System)"=21964, "CAN-Task (Blockdiagrammkonstante)"=3471, "CAN-Task (Klassisch)"=3470, "CAN-Task (Modern)"=21789, "CAN-Task (System)"=21963, "Case-Struktur"=2001, "Cluster (Klassisch)"=3400, "Cluster (Modern)"=21607, "Cluster nach Array"=1169, "Cluster-Array erstellen"=2047, "Cluster-Array indizieren und bündeln"=2056, "Cluster-Konstante"=2071, "Code-Interface-Knoten"=2050, "Cosecans"=1204, "Cosecans Hyperbolicus"=23053, "Cosinus"=1201, "Cosinus Hyperbolicus"=1215, "Cotangens"=1205, "Cotangens Hyperbolicus"=23055, "CPU-Informationen"=24130, "DAQ-Kanal (Traditionell) (Blockdiagrammkonstante)"=2085, "DAQ-Kanal (Traditionell) (Klassisch)"=3320, "DAQ-Kanal (Traditionell) (Modern)"=21733, "DAQmx - Analog-Trigger-Quelle (Blockdiagrammkonstante)"=2119, "DAQmx - Analog-Trigger-Quelle (Klassisch)"=3336, "DAQmx - Analog-Trigger-Quelle (Modern)"=21774, "DAQmx - Analog-Trigger-Quelle (System)"=21951, "DAQmx - Globaler Kanal (Blockdiagrammkonstante)"=3430, "DAQmx - Globaler Kanal (Klassisch)"=3443, "DAQmx - Globaler Kanal (Modern)"=21770, "DAQmx - Globaler Kanal (System)"=21957, "DAQmx - Physikalischer Kanal (Blockdiagrammkonstante)"=2118, "DAQmx - Physikalischer Kanal (Klassisch)"=3335, "DAQmx - Physikalischer Kanal (Modern)"=21777, "DAQmx - Physikalischer Kanal (System)"=21954, "DAQmx-Anschluss (Blockdiagrammkonstante)"=2117, "DAQmx-Anschluss (Klassisch)"=3319, "DAQmx-Anschluss (Modern)"=21781, "DAQmx-Anschluss (System)"=21955, "DAQmx-Gerätename (Blockdiagrammkonstante)"=2093, "DAQmx-Gerätename (Klassisch)"=3318, "DAQmx-Gerätename (Modern)"=21773, "DAQmx-Gerätename (System)"=21950, "DAQmx-Skalierungsname (Blockdiagrammkonstante)"=2116, "DAQmx-Skalierungsname (Klassisch)"=3317, "DAQmx-Skalierungsname (Modern)"=21775, "DAQmx-Skalierungsname (System)"=21952, "DAQmx-Switch (Blockdiagrammkonstante)"=2121, "DAQmx-Switch (Klassisch)"=3337, "DAQmx-Switch (Modern)"=21776, "DAQmx-Switch (System)"=21953, "DAQmx-Task-Name (Blockdiagrammkonstante)"=3434, "DAQmx-Task-Name (Klassisch)"=3442, "DAQmx-Task-Name (Modern)"=21778, "DAQmx-Task-Name (System)"=21959, "DataSocket-Referenz"=3417, "DataSocket: Lesen"=1086, "DataSocket: Schließen"=1085, "DataSocket: Schreiben"=1087, "DataSocket: Öffnen"=1084, "Datei lesen"=1407, "Datei schließen"=8052, "Datei schließen (veraltet)"=1405, "Datei schreiben"=1408, "Datei öffnen"=1403, "Datei- und Programmtyp"=1434, "Datei- und Programmtyp ermitteln"=8066, "Datei- und Programmtyp festlegen"=8077, "Datei-/Verzeichnis-Info"=8082, "Datei-/Verzeichnis-Info (veraltet)"=1413, "Dateidialog"=8058, "Dateidialog (veraltet)"=8081, "Dateigröße ermitteln"=8063, "Dateigröße festlegen"=8074, "Dateipfad-Anzeigeelement (Klassisch)"=3204, "Dateipfad-Anzeigeelement (Modern)"=21731, "Dateipfad-Bedienelement (Klassisch)"=3203, "Dateipfad-Bedienelement (Modern)"=21730, "Dateipfad-Bedienelement (System)"=21922, "Dateiposition ermitteln"=8062, "Dateiposition festlegen"=8073, "Dateipuffer leeren"=8059, "Dateipuffer leeren (veraltet)"=1406, "Daten serialisieren"=1164, "Daten-Cache-Größe"=24132, "Datenprotokoll lesen"=8069, "Datenprotokoll schreiben"=8079, "Datenprotokolldatei (Referenz)"=3402, "Datenträger-Info"=1414, "Datenträger-Info lesen"=8067, "Datenwertreferenz löschen"=2409, "Datum-/Zeit-String lesen"=1600, "Datum/Zeit formatieren"=8100, "Datum/Zeit in Sekunden ermitteln"=1303, "Datum/Zeit nach Sekunden"=1308, "Dekrementieren"=1058, "DevClear"=1961, "DevClearList"=1962, "Dezimal-String nach Zahl"=1184, "Dezimalzeichen gleich?"=23064, "Dezimalziffer?"=1119, "Diagrammdeaktivierungsstruktur"=2054, "Dialogfeld mit einer Schaltfläche"=1340, "Dialogfeld mit zwei Schaltflächen"=1341, "Digitaldaten (Klassisch)"=3210, "Digitaldaten (Modern)"=21216, "Digitaler Signalverlaufsgraph (Klassisch)"=3511, "Digitaler Signalverlaufsgraph (Modern)"=21718, "Dividieren"=1053, "Dividieren (mit Fehleranschlüssen)"=3918, "Dlg Horiz. Bildlaufleiste"=21905, "Dlg Numerisch 1"=2100, "Dlg Numerisch 2"=3006, "Dlg String"=2110, "Dlg Vert. Bildlaufleiste"=21906, "Drehknopf (Klassisch)"=3005, "Drehknopf (Modern)"=21000, "Drehregler (Klassisch)"=3050, "Drehregler (Modern)"=21732, "Drehspulinstrument (Klassisch)"=3030, "Drehspulinstrument (Modern)"=21008, "Dreieck (abwärts)"=3623, "Dreieck (aufwärts)"=3622, "Dreieck (links)"=3620, "Dreieck (rechts)"=3621, "Dreiecksrelief (abwärts)"=3615, "Dreiecksrelief (aufwärts)"=3614, "Dreiecksrelief (links)"=3612, "Dreiecksrelief (rechts)"=3613, "Druckbar?"=1124, "Druckschalter"=21001, "Druckschalter (rechteckig)"=3119, "Druckschalter (rechteckig) (Profil)"=3113, "Druckschalter (rund)"=3118, "Druckschalter (rund) (Profil)"=3112, "Drucktank (flach)"=3075, "Drucktank (Klassisch)"=3070, "Drucktank (Modern)"=21751, "Drucktank (schattiert)"=21753, "Dynamische FPGA-Schnittstellen-Umwandlung"=5690, "Eigenschaftsknoten"=1920, "Ein Element aus Stream auslesen"=23797, "Ein Element in Stream schreiben"=23798, "Einfacher horiz. Schieber"=3003, "Einfacher String"=2115, "Einfacher vert. Schieber"=3002, "Einfaches numerisches Feld"=2900, "Einheit umrechnen"=2059, "Element am Anfang einfügen"=9129, "Element aus Queue entfernen"=9113, "Element einfügen"=9111, "Element einfügen (verlustbehaftet)"=9130, "Elementarladung (C)"=23517, "Elementreferenz"=3419, "Elternmethode aufrufen"=2354, "Empfangen"=1974, "Empfangsendpunkt für Netzwerk-Stream erstellen"=23811, "EnableLocal"=1963, "EnableRemote"=1964, "Enum (Klassisch)"=3023, "Enum (Modern)"=21605, "Enum (System)"=3062, "Enum-Konstante"=2090, "EOF"=1410, "Ereignis-Callback (Referenz)"=3435, "Ereignis-Callback registrieren"=2078, "Ereignisdatenknoten"=2102, "Ereignisregistrierung aufheben"=2076, "Ereignisstruktur"=2052, "Ersten String suchen"=1532, "Erster Aufruf?"=1083, "Exklusiv-NICHT-ODER"=1073, "Exklusiv-ODER"=1063, "Exponential"=1211, "Exponential (Arg) -1"=1222, "FALSE-Konstante"=2006, "Farbfeld"=3013, "Farbfeld mit dünnem Rahmen"=2905, "Farbfeld mit Rahmen (Klassisch)"=3008, "Farbfeld mit Rahmen (Modern)"=21019, "Farbfeldkonstante"=2120, "Farbiges Rechteck (Fehler?)"=3625, "Farbrampe"=3022, "Fehler zusammenfassen"=2147, "Fehler-Ringkonstante"=2039, "Festkomma in Integer umwandeln"=5566, "Festkomma-Überlaufzustand einschließen"=5564, "Festkomma-Überlaufzustand entfernen"=5563, "Festkomma-Überlaufzustand löschen"=5562, "Festkommakomponenten erfassen"=11163, "Festkommaüberlauf?"=5565, "FieldPoint-I/O-Kanal (Blockdiagrammkonstante)"=3440, "FieldPoint-I/O-Kanal (Klassisch)"=3439, "FieldPoint-I/O-Kanal (Modern)"=21784, "FIFO (Referenz)"=3474, "FindLstn"=1965, "FindRQS"=1966, "Flache Sequenzstruktur"=2069, "Fließkantenrelief (horizontal)"=3633, "Fließkantenrelief (vertikal)"=3634, "For-Schleife"=2002, "Formelknoten"=2004, "FPGA-Referenz nach Session"=2322, "Freie Beschriftung"=2321, "Frontpanel-Aktivität generieren"=1329, "Förderband"=3827, "Für Ereignisse registrieren"=2065, "Gabelung"=2194, "Gerät lesen"=1432, "Gerät schreiben"=1431, "Gerät öffnen"=1430, "Gerätereferenz"=3405, "Gerätsteuerung/Status"=1433, "Gestapelte Sequenzstruktur"=2000, "Gleich 0?"=1113, "Gleich?"=1102, "Globale Variable"=2060, "GPIB: Initialisierung"=1957, "GPIB: Lesen"=1951, "GPIB: Schreiben"=1950, "GPIB: Serielles Pollen"=1955, "GPIB: Status"=1959, "GPIB: Trigger"=1953, "GPIB: Verschiedenes"=1956, "GPIB: Warten"=1958, "GPIB: Zurücksetzen"=1954, "Grafikring (Klassisch)"=3015, "Grafikring (Modern)"=21602, "Grafikring (System)"=21925, "Gravitationskonstante (N m2/kg2)"=23519, "Größen-Handle"=1603, "Größer als 0?"=1117, "Größer oder gleich 0?"=1114, "Größer oder gleich?"=1103, "Größer?"=1110, "Heizkessel"=3829, "Hexadezimal-String nach Zahl"=1185, "Hexadezimalziffer?"=1123, "Hilfefenster steuern"=1353, "Hinzufügen (mit Fehleranschlüssen)"=3915, "Horiz. Linie"=3821, "Horiz. Rohrleitung (flach)"=3810, "Horiz. Rohrleitung (schattiert)"=3710, "Horiz. Rundbox"=3636, "Horizontaler Trennbalken (Klassisch)"=21863, "Horizontaler Trennbalken (System)"=21865, "ID des aktuellen Prozessors"=24131, "IMAQ-Session"=3415, "Immer kopieren"=2400, "Implikation"=1080, "In Array einfügen"=3911, "In Binärdatei schreiben"=8078, "In Datei formatieren"=2083, "In Datei suchen"=2082, "In Großbuchstaben"=1188, "In Kleinbuchstaben"=1189, "In OLE-Variant"=8002, "In String formatieren"=2081, "In String suchen"=2080, "In Textdatei schreiben"=8080, "In XML konvertieren"=8400, "Inkrementieren"=1057, "Inline-C-Knoten"=2104, "Inplace-Elementstruktur"=2360, "Integer in Festkomma umwandeln"=5567, "Intensitätsdiagramm (Klassisch)"=3509, "Intensitätsdiagramm (Modern)"=21719, "Intensitätsgraph (Klassisch)"=3510, "Intensitätsgraph (Modern)"=21720, "Intervall #1"=3073, "Intervall #2"=21755, "IP nach String"=1710, "IrDA-Netzwerkverbindung (Referenz)"=3450, "IrDA: Auf Listener warten"=9143, "IrDA: Geräte suchen"=9141, "IrDA: Lesen"=9145, "IrDA: Listener erzeugen"=9140, "IrDA: Schreiben"=9146, "IrDA: Verbindung herstellen"=9142, "IrDA: Verbindung schließen"=9144, "IVI Session löschen"=8103, "Kehrwert"=1059, "Kehrwert von e"=23511, "Kehrwert von Pi"=23507, "Kein Pfad (Konstante)"=23524, "Keine Referenz (Konstante)"=23526, "Keine Umgebungsvariable"=23527, "Keine Zahl/Kein Pfad/Keine Referenz?"=1128, "Kippschalter"=21002, "Kippschalter (vertikal)"=21740, "Klassenbezeichner-Konstante"=2094, "Kleiner als 0?"=1118, "Kleiner oder gleich 0?"=1115, "Kleiner oder gleich?"=1104, "Kleiner?"=1111, "Knoten zum Aufruf externer Bibliotheken"=2062, "Kombinationsfeld (Klassisch)"=3304, "Kombinationsfeld (Modern)"=21604, "Kombinationsfeld (System)"=21917, "Kombinationsfeldkonstante"=2088, "Komplex nach polar"=1045, "Komplex nach Re/Im"=1044, "Komplex-Konjugierte"=1048, "Kompressor"=3832, "Konstruktorknoten"=3904, "Kopieren"=8053, "Kopieren (veraltet)"=1416, "Kreis"=3605, "Kreisförmiges Relief"=3603, "Kreuzung"=2197, "LabVIEW beenden"=1352, "LabVIEW-Objekt"=3457, "Laufzeitklasse erhalten"=8018, "Leak Variant Value Reference"=2410, "LED (rechteckig) (Klassisch)"=3121, "LED (rechteckig) (Modern)"=21013, "LED (rund) (Klassisch)"=3120, "LED (rund) (Modern)"=21012, "LED-Schalter"=3116, "Leerer Pfad (Konstante)"=23523, "Leerer String (Konstante)"=23503, "Leerer String/Pfad?"=1112, "Leeres Array?"=23063, "Leuchte (rechteckig)"=3105, "Leuchte (rund)"=3104, "Lexikalische Klasse"=1126, "Lichtgeschwindigkeit im Vakuum (m/s)"=23518, "Linie (dick)"=3629, "Linie (dünn)"=3626, "Linie (vertieft) (System)"=3632, "Linie (vertieft, dick)"=3630, "Linie (vertieft, dünn)"=3627, "Linie mit Pfeil (dick)"=3631, "Linie mit Pfeil (dünn)"=3628, "Listenfeld (Klassisch)"=21806, "Listenfeld (Modern)"=21792, "Listenfeld (System)"=21805, "Listenfeldsymbol-Ringkonstante"=2038, "Logarithmus zur Basis 10"=1210, "Logarithmus zur Basis 10 von e"=23512, "Logarithmus zur Basis 2"=1225, "Logarithmus zur Basis x"=1224, "Logischer IVI-Name (Blockdiagrammkonstante)"=3420, "Logischer IVI-Name (Klassisch)"=3414, "Logischer IVI-Name (Modern)"=21736, "Logisches Verschieben"=1081, "Lokale Variable"=2061, "Löschen"=8056, "Löschen (veraltet)"=1417, "Mantisse und Exponent"=1150, "Maschinengenauigkeit"=23528, "MathScript-Aufruf über Referenzknoten"=3906, "MathScript-Knoten"=2357, "MATLAB-Skript"=9020, "Matrix entpacken"=23000, "Matrix erstellen"=8500, "Matrix transponieren"=8509, "Matrixdiagonale festlegen"=8504, "Matrixdiagonale lesen"=8501, "Matrixelemente festlegen"=8505, "Matrixelemente lesen"=8502, "Matrixgröße"=8507, "Matrixgröße ändern"=8508, "Max & Min"=1108, "Max. & Min. von Array"=1907, "Mehrere Elemente aus Stream auslesen"=23803, "Mehrere Elemente in Stream schreiben"=23804, "Mehrfacharithmetik"=2200, "Mehrsegmentrohr"=23780, "Mehrspaltiges Listenfeld (Klassisch)"=21799, "Mehrspaltiges Listenfeld (Modern)"=21791, "Mehrspaltiges Listenfeld (System)"=21798, "Melder anfordern"=9101, "Melder freigeben"=9102, "Melderreferenz"=3423, "Melderstatus lesen"=9103, "Meldung abbrechen"=9107, "Meldung senden"=9104, "Menü-Popup-Ring"=3017, "Menüauswahl abfragen"=9001, "Menüleiste des aktuellen VIs"=9000, "Menüpunkt-Info lesen"=9005, "Menüpunkte einfügen"=9003, "Menüpunkte löschen"=9004, "Menüpunkteinstellungen"=9006, "Menüreferenz"=3413, "Menüring (Klassisch)"=3018, "Menüring (Modern)"=21600, "Menüverknüpfung abfragen"=9007, "Messleiste (horizontal)"=21106, "Messleiste (vertikal)"=21107, "Methodenknoten"=3900, "Mischsignalgraph"=21721, "Mit Potenz von 2 multiplizieren"=1074, "Molare Gas-Konstante (J/(mol K))"=23522, "Motion-Ressource (Blockdiagrammkonstante)"=3449, "Motion-Ressource (Klassisch)"=3448, "Motion-Ressource (Modern)"=21787, "Motor (flach)"=3820, "Motor (schattiert)"=3720, "Multifrequenzstruktur"=2199, "Multiplizieren"=1052, "Multiplizieren (mit Fehleranschlüssen)"=3917, "Muster suchen"=1535, "Nach allgemeinerer Klasse"=8017, "Nach Byte-Integer"=1140, "Nach Festkomma"=5561, "Nach Fließkommawert (doppelte Genauigkeit)"=1147, "Nach Fließkommawert (einfache Genauigkeit)"=1146, "Nach Fließkommawert (erweitert)"=1149, "Nach Komplex (doppelte Genauigkeit)"=1152, "Nach Komplex (einfache Genauigkeit)"=1151, "Nach Komplex (höchste Genauigkeit)"=1154, "Nach links rotieren (mit Übertrag)"=1606, "Nach Long-Integer"=1142, "Nach Namen aufschlüsseln"=2058, "Nach Namen bündeln"=2057, "Nach Quad-Integer"=1155, "Nach rechts rotieren (mit Übertrag)"=1607, "Nach Sonden-String"=2413, "Nach spezifischerer Klasse"=8016, "Nach Variant"=8201, "Nach vorzeichenlosen Byte-Integer"=1143, "Nach vorzeichenlosen Long-Integer"=1145, "Nach vorzeichenlosen Quad-Integer"=1156, "Nach vorzeichenlosen Wort-Integer"=1144, "Nach Wert durchsuchen"=1534, "Nach Wort-Integer"=1141, "Nach Zeitstempel"=5560, "Natürlicher Logarithmus"=1209, "Natürlicher Logarithmus (Arg +1)"=1221, "Natürlicher Logarithmus von 10"=23513, "Natürlicher Logarithmus von 2"=23514, "Natürlicher Logarithmus von Pi"=23508, "Negativ unendlich"=23509, "Negieren"=1069, "Neue Datei"=1404, "Neue Datenwertreferenz"=2408, "Neue IVI-Session"=8102, "Neues Verzeichnis"=1402, "Neues VI"=8014, "Neues VI-Objekt"=8015, "NICHT"=1064, "Nicht darstellbares Zeichen?"=1125, "Nicht-ODER"=1072, "Nicht-UND"=1071, "Numerische Konstante"=2005, "Numerisches Anzeigeelement (Klassisch)"=3001, "Numerisches Anzeigeelement (Modern)"=21004, "Numerisches Bedienelement (Klassisch)"=3000, "Numerisches Bedienelement (Modern)"=21003, "Numerisches Bedienelement (System)"=21919, "Occurrence (Referenz)"=3406, "Occurrence erzeugen"=1700, "Occurrence festlegen"=1702, "ODER"=1062, "ODER (Array-Elemente)"=1910, "Offener Tank (flach) (Klassisch)"=21752, "Offener Tank (schattiert) (Klassisch)"=3074, "OK-Schaltfläche (Modern)"=21738, "OK-Schaltfläche (System)"=3130, "Oktal-String nach Zahl"=1186, "Oktalziffer?"=1129, "OLE-Variant"=3150, "Online-Hilfe steuern"=1355, "Optionsfeld (rechteckig)"=3107, "Optionsfeld (rund)"=3106, "Optionsfeld (System)"=3133, "Optionsfelder (Klassisch)"=22003, "Optionsfelder (Modern)"=22001, "Optionsfelder (System)"=22002, "Ordner anzeigen"=8083, "Ordner erstellen"=8055, "Paketmatrix"=23001, "PassControl"=1968, "Peek-Operation verarbeiten"=1604, "Pfad des aktuellen VIs"=1426, "Pfad erstellen"=1419, "Pfad nach Array aus Strings"=1423, "Pfad nach String"=1077, "Pfad zerlegen"=1420, "Pfadkonstante"=2009, "Pfadtyp"=1421, "Pfeil (Abwärts)"=3824, "Pfeil (aufwärts)"=3823, "Pfeil (links)"=3826, "Pfeil (rechts)"=3825, "Pi"=23504, "Pi geteilt durch 2"=23506, "Pi multipliziert mit 2"=23505, "PixMap"=3505, "PixMap (Warnung: gefährlich)"=3507, "Planck-Konstante (J/Hz)"=23516, "Plattform: Flache Rechteck-Schaltfläche"=3134, "Plugin-Steuerung"=21820, "Poke-Operation verarbeiten"=1605, "Polar nach komplex"=1047, "Polar nach Re/Im"=23061, "Position im Datenprotokoll ermitteln"=8061, "Position im Datenprotokoll festlegen"=8072, "Positiv unendlich"=23515, "Potenz von 10"=1212, "Potenz von 2"=1223, "PPoll"=1969, "PPollConfig"=1970, "PPollUnconfig"=1971, "Pulldown-Menüring"=3061, "Pumpe (links) (flach)"=3813, "Pumpe (links) (schattiert)"=3713, "Pumpe (rechts) (flach)"=3819, "Pumpe (rechts) (schattiert)"=3719, "Quadrat"=23059, "Quadratwurzel"=1060, "Queue anfordern"=9108, "Queue freigeben"=9109, "Queue leeren"=9114, "Queue-Referenz"=3424, "Queue-Status lesen"=9110, "Quotient und Rest"=1056, "Rahmen"=3608, "RcvRespMsg"=1972, "Re/Im nach komplex"=1046, "Re/Im nach polar"=23060, "ReadStatus"=1973, "ReceiveSetup"=1975, "Rechteck"=3602, "Rechteckschaltfläche"=3103, "Referenz nach Pfad"=1424, "Referenz nach Session"=2306, "Referenz schließen"=8011, "Regel- und Simulationsschleife"=2099, "Registerkartenelement (Klassisch)"=3330, "Registerkartenelement (Modern)"=3332, "Registerkartenelement (System)"=3331, "Registrierung für Sitzung entfernen"=2320, "Registrierungssession"=2319, "Reliefrahmen"=3606, "ResetSys"=1976, "Ressourcen-Index"=1088, "Rohrknie (links, abwärts) (flach)"=3811, "Rohrknie (links, abwärts) (schattiert)"=3711, "Rohrknie (links, aufwärts) (flach)"=3708, "Rohrknie (links, aufwärts) (flach) 1"=3808, "Rohrknie (rechts, abwärts) (flach)"=3817, "Rohrknie (rechts, abwärts) (schattiert)"=3717, "Rohrknie (rechts, aufwärts) (flach)"=3814, "Rohrknie (rechts, aufwärts) (schattiert)"=3714, "Rotationsverteiler"=3830, "Rotieren"=1082, "RT-FIFO erstellen"=24000, "RT-FIFO lesen"=24001, "RT-FIFO löschen"=24003, "RT-FIFO schreiben"=24002, "Rundinstrument (Klassisch)"=3040, "Rundinstrument (Modern)"=21009, "Rundschaltfläche"=3102, "Rydberg-Konstante (1/m)"=23521, "Rückkopplungsknoten"=2353, "Schalter (horizontal)"=3108, "Schalter (vertikal)"=3109, "Schaltfläche (rechteckig)"=3101, "Schaltfläche (rund)"=3100, "Schieber (horizontal) (Klassisch)"=3010, "Schieber (horizontal) (System)"=21904, "Schieber (horizontal, gefüllt) (Klassisch)"=3012, "Schieber (horizontal, gefüllt) (Modern)"=21100, "Schieber (vertikal) (System)"=21903, "Schieber (vertikal, gefüllt) (Klassisch)"=3009, "Schieber (vertikal, gefüllt) (Modern)"=21014, "Schieber mit Knopf (vertikal)"=3004, "Schieber mit Zeiger (horizontal) (Klassisch)"=3011, "Schieber mit Zeiger (horizontal) (Modern)"=21101, "Schieber mit Zeiger (horizontal) (System)"=21902, "Schieber mit Zeiger (vertikal) (Klassisch)"=3007, "Schieber mit Zeiger (vertikal) (Modern)"=21017, "Schieber mit Zeiger (vertikal) (System)"=21901, "Schiebeschalter"=21011, "Schiebeschalter (horizontal)"=3114, "Schiebeschalter (vertikal) (Klassisch)"=3115, "Schiebeschalter (vertikal) (Modern)"=21741, "Schwellwert (1D-Array)"=1909, "Secans"=1203, "Secans Hyperbolicus"=23054, "Sekunden nach Datum/Zeit"=1309, "SendCmds"=1978, "SendDataBytes"=1979, "Sendeendpunkt für Netzwerk-Stream erstellen"=23810, "Senden"=1977, "SendIFC"=1980, "SendList"=1981, "SendLLO"=1982, "SendSetup"=1983, "Serialisierte Daten nach Variant"=8202, "Serialisiertes benutzerdef. Referenz-Tag (Klassisch)"=3454, "Serialisiertes benutzerdef. Referenz-Tag (Modern)"=21747, "Session nach Referenz"=2307, "SetRWLS"=1984, "SetTimeOut"=1985, "Signale trennen"=2351, "Signale zusammenfassen"=2350, "Signalverlauf erstellen"=2066, "Signalverlaufsattribut entfernen"=8209, "Signalverlaufsattribut ermitteln"=8208, "Signalverlaufsattribut festlegen"=8207, "Signalverlaufsdiagramm"=21010, "Signalverlaufsdiagramm (Klassisch)"=3501, "Signalverlaufsdiagramm (Modern)"=21717, "Signalverlaufsgraph (Klassisch)"=3504, "Signalverlaufsgraph (Modern)"=21703, "Signalverlaufskomponenten lesen"=2067, "Sinc"=1227, "Sinus"=1200, "Sinus Hyperbolicus"=1214, "Sinus und Cosinus"=1220, "Speicherfreigabe anfordern"=1610, "Standardverzeichnis"=1427, "Statische VI-Referenz"=2084, "Status des Hilfefensters lesen"=1354, "Stopp"=1350, "Stopp-Schaltfläche"=21230, "Stopp-Schaltfläche (rechteckig)"=3128, "Stopp-Schaltfläche (rund)"=3127, "Stream beenden"=23807, "Stream erstellen"=23796, "Stream leeren"=23808, "Stream prüfen und verknüpfen"=23805, "Stream starten"=23806, "Stream verknüpfen"=23793, "Stream-Endpunkt entfernen"=23794, "Stream-Verknüpfung aufheben"=23795, "String deserialisieren"=1165, "String durchsuchen und teilen"=1538, "String nach Byte-Array"=1608, "String nach IP"=1711, "String nach Pfad"=1078, "String nach Token durchsuchen"=8101, "String nach Umgebungsvariable"=1830, "String rotieren"=1536, "String suchen und ersetzen"=3914, "String umkehren"=1537, "String-Anzeigeelement (Klassisch)"=3201, "String-Anzeigeelement (Modern)"=21702, "String-Array indizieren"=1531, "String-Bedienelement (Klassisch)"=3200, "String-Bedienelement (Modern)"=21701, "String-Bedienelement (System)"=21920, "String-Konstante"=2007, "String-Länge"=1502, "Stringarray sortieren"=23065, "Strings verknüpfen"=2040, "Subtrahieren"=1051, "Subtrahieren (mit Fehleranschlüssen)"=3916, "Suchen"=1409, "T-Stück (abwärts) (flach)"=3818, "T-Stück (abwärts) (schattiert)"=3718, "T-Stück (aufwärts) (flach)"=3812, "T-Stück (aufwärts) (schattiert)"=3712, "T-Stück (links) (flach)"=3809, "T-Stück (links) (schattiert)"=3709, "T-Stück (rechts) (flach)"=3815, "T-Stück (rechts) (schattiert)"=3715, "Tabelle (Klassisch)"=21796, "Tabelle (Modern)"=21790, "Tabelle (System)"=21797, "Tabellen-String nach Array"=1539, "Tabulatorkonstante"=23502, "Tag-Attributring"=2063, "Tangens"=1202, "Tangens Hyperbolicus"=1216, "Tank (horizontal)"=3071, "Tank (Klassisch)"=3020, "Tank (Modern)"=21006, "TCP-Netzwerkverbindung (Referenz)"=3407, "TCP: Auf Listener warten"=1712, "TCP: Lesen"=1716, "TCP: Lesen (Flex.)"=1720, "TCP: Lesen (Strings)"=1718, "TCP: Listener erstellen"=1717, "TCP: Schreiben"=1714, "TCP: Schreiben (Flex.)"=1721, "TCP: Schreiben (Strings)"=1719, "TCP: Verbindung herstellen"=1715, "TCP: Verbindung schließen"=1713, "TDMS Close"=24113, "TDMS Defragment"=24119, "TDMS Flush"=24117, "TDMS Get Properties"=24115, "TDMS List Contents"=24116, "TDMS Open"=24112, "TDMS Read"=24111, "TDMS Refnum To File ID"=24120, "TDMS Set Properties"=24114, "TDMS Write"=24110, "TDMS Write IP"=24118, "TDMS: Datei"=3477, "Teil-Array"=2044, "Teil-Array ersetzen"=3910, "Teil-String"=1503, "Teil-String ersetzen"=3913, "Temporäres Verzeichnis"=1435, "TestSRQ"=1986, "TestSys"=1987, "Text nach UTF-8"=23066, "Text- & Grafikring (Klassisch)"=3016, "Text- & Grafikring (Modern)"=21603, "Text-Schaltfläche"=21015, "Textring (Blockdiagrammkonstante)"=2008, "Textring (Klassisch)"=3014, "Textring (Modern)"=21601, "Textring (System)"=3060, "Thermometer (Klassisch)"=3021, "Thermometer (Modern)"=21007, "Timer-Wert (ms)"=1300, "Trennbalken (horizontal)"=21861, "Trennbalken (vertikal)"=21860, "Trennschalter"=21020, "Trichter 1"=21754, "Trichter 2"=3072, "Trigger"=1988, "TriggerList"=1989, "TRUE/FALSE-String anhängen"=1511, "TRUE/FALSE-String suchen"=1533, "Typ erzwingen"=2402, "Typumwandlung"=1166, "UDP-Netzwerkverbindung (Referenz)"=3418, "UDP: Lesen"=1724, "UDP: Multicast öffnen"=1727, "UDP: Schließen"=1726, "UDP: Schreiben"=1725, "UDP: Öffnen"=1723, "Umgebungsvariable"=23778, "Umgebungsvariable nach String"=1831, "Umgebungsvariablenelement (Klassisch)"=3472, "Umgebungsvariablenelement (Modern)"=21814, "Umgebungsvariablenkonstante"=3473, "Umschalter (horizontal) (Klassisch)"=3110, "Umschalter (horizontal) (Modern)"=21700, "Umschalter (vertikal) (Klassisch)"=3111, "Umschalter (vertikal) (Modern)"=21005, "Unbitpack von Array"=3136, "UND"=1061, "UND (Array-Elemente)"=1911, "Ungleich 0?"=1116, "Ungleich?"=1105, "Unleak Variant Value Reference"=2411, "Untermatrix festlegen"=8506, "Untermatrix lesen"=8503, "Unterpanel"=21810, "Unterpanel (klassisch)"=21811, "Unterpanel (System)"=21823, "UTF-8 nach Text"=23067, "Variable auslesen (mit Timeout)"=23786, "Variable direkt lesen"=23785, "Variable direkt schreiben"=23788, "Variable lesen"=23781, "Variable lesen (Scan)"=23784, "Variable schreiben"=23782, "Variable schreiben (mit Timeout)"=23789, "Variable schreiben (Scan)"=23787, "Variablen-Container suchen"=23802, "Variablenklassenbezeichner-Konstante"=2106, "Variablenkonfiguration"=3475, "Variablenname (Konstante)"=3478, "Variablenverbindung beenden"=23783, "Variablenverbindung herstellen"=23779, "Variablenverbindung herstellen und prüfen"=23790, "Variablenverbindung im Hintergrund herstellen"=23791, "Variant"=3310, "Variant nach Daten"=8003, "Variant nach serialisierte Daten"=8203, "Variant wieder zusammensetzen (Warnung: gefährlich)"=2405, "Variant zerlegen"=2404, "Variantattribut entfernen"=8206, "Variantattribut ermitteln"=8205, "Variantattribut festlegen"=8204, "Vektorwerte austauschen"=1912, "Ventil (Abwärtsbogen) (flach)"=3707, "Ventil (Abwärtsbogen) (schattiert)"=21767, "Ventil (Abwärtsbogen) (Umriss)"=3807, "Ventil (Aufwärtsbogen) (flach)"=3703, "Ventil (Aufwärtsbogen) (schattiert)"=21763, "Ventil (Aufwärtsbogen) (Umriss)"=3803, "Ventil (Linksbogen) (flach)"=3701, "Ventil (Linksbogen) (schattiert)"=21761, "Ventil (Linksbogen) (Umriss)"=3801, "Ventil (Rechtsbogen) (flach)"=3705, "Ventil (Rechtsbogen) (schattiert)"=21765, "Ventil (Rechtsbogen) (Umriss)"=3805, "Ventil (rechtwinklig, abwärts) (flach)"=3706, "Ventil (rechtwinklig, abwärts) (schattiert)"=21766, "Ventil (rechtwinklig, abwärts) (Umriss)"=3806, "Ventil (rechtwinklig, aufwärts) (flach)"=3702, "Ventil (rechtwinklig, aufwärts) (schattiert)"=3802, "Ventil (rechtwinklig, aufwärts) (Umriss)"=21762, "Ventil (rechtwinklig, links) (flach)"=3700, "Ventil (rechtwinklig, links) (schattiert)"=21760, "Ventil (rechtwinklig, links) (Umriss)"=3800, "Ventil (rechtwinklig, rechts) (flach)"=3704, "Ventil (rechtwinklig, rechts) (schattiert)"=21764, "Ventil (rechtwinklig, rechts) (Umriss)"=3804, "Ventil prüfen"=3833, "Vereinigung"=2195, "Verlaufsanzeige (horizontal) (Modern)"=21102, "Verlaufsanzeige (horizontal) (System)"=21910, "Verlaufsanzeige (vertikal) (Modern)"=21104, "Verlaufsanzeige (vertikal) (System)"=21909, "Verschieben"=8068, "Verschieben (veraltet)"=1415, "Verschobene Daten ermitteln"=9154, "Vert. Linie"=3822, "Vert. Rohrleitung (flach)"=3816, "Vert. Rohrleitung (schattiert)"=3716, "Vertikaler Trennbalken (Klassisch)"=21862, "Vertikaler Trennbalken (System)"=21864, "Verzeichnis auflisten"=1418, "VI-Bibliothek"=1425, "VI-Objektreferenz öffnen"=8013, "VI-Referenz"=3422, "VI-Referenz öffnen"=8010, "VI-Server-Referenz"=2091, "Viereckiges Relief (Klassisch)"=3600, "Viereckiges Relief (Modern)"=3637, "Viereckiges Relief (runde Ecken)"=3609, "VISA-Referenz nach Session"=2300, "VISA-Ressourcenname"=3421, "VISA-Ressourcenname (Klassisch)"=3409, "VISA-Ressourcenname (Modern)"=21737, "VISA: Adresse freigeben"=1933, "VISA: Adresse zuweisen"=1932, "VISA: Auf Ereignis warten"=1943, "VISA: Bereich lesen (16)"=1948, "VISA: Bereich lesen (32)"=1991, "VISA: Bereich lesen (64)"=2144, "VISA: Bereich lesen (8)"=1946, "VISA: Bereich schreiben (16)"=1949, "VISA: Bereich schreiben (32)"=1992, "VISA: Bereich schreiben (64)"=2145, "VISA: Bereich schreiben (8)"=1947, "VISA: Ereignis aktivieren"=1942, "VISA: Ereignis deaktivieren"=1940, "VISA: Ereignis verwerfen"=1941, "VISA: GPIB sendet IFC"=2318, "VISA: GPIB steuert ATN"=2316, "VISA: GPIB steuert REN"=2304, "VISA: GPIB-Befehl"=2315, "VISA: GPIB-Durchgangssteuerung"=2317, "VISA: Hilfssignal anfordern"=2310, "VISA: I/O-Puffer entleeren"=2302, "VISA: I/O-Puffergröße festlegen"=2301, "VISA: In Datei lesen"=2313, "VISA: Interrupt anfordern"=2309, "VISA: Lesen"=1925, "VISA: Peek (16)"=1934, "VISA: Peek (32)"=1995, "VISA: Peek (64)"=2142, "VISA: Peek (8)"=1938, "VISA: Poke (16)"=1935, "VISA: Poke (32)"=1996, "VISA: Poke (64)"=2143, "VISA: Poke (8)"=1939, "VISA: Ressource suchen"=1923, "VISA: Schließen"=1922, "VISA: Schreiben"=1926, "VISA: Speicher freigeben"=1998, "VISA: Speicher reservieren"=1997, "VISA: Speicher reservieren (Ex)"=2146, "VISA: Sperre aufheben"=1994, "VISA: Sperren"=1993, "VISA: Statusinformation"=1924, "VISA: STB lesen"=1928, "VISA: Trigger freigeben"=2312, "VISA: Trigger freigeben 1"=1929, "VISA: Trigger zuweisen"=2311, "VISA: USB-Steuerung (Ausgang)"=2087, "VISA: USB-Steuerung (Eingang)"=2086, "VISA: Verschieben"=2303, "VISA: Von Datei schreiben"=2314, "VISA: VXI-Befehl oder -Abfrage"=2305, "VISA: Wert lesen (16)"=1930, "VISA: Wert lesen (32)"=1944, "VISA: Wert lesen (64)"=2140, "VISA: Wert lesen (8)"=1936, "VISA: Wert schreiben (16)"=1931, "VISA: Wert schreiben (32)"=1945, "VISA: Wert schreiben (64)"=2141, "VISA: Wert schreiben (8)"=1937, "VISA: Zurücksetzen"=1927, "VISA: Öffnen"=2308, "VISA: Öffnen (alt)"=1921, "Vorschau für Queue-Element"=9112, "Vorzeichen"=1049, "Wagenrücklauf-Konstante"=23500, "WaitSRQ"=1990, "Warten (ms)"=1302, "Wert formatieren"=1512, "Werte austauschen"=2401, "Wertebereich prüfen und erzwingen"=1127, "While-Schleife 1"=2003, "While-Schleife 2"=2352, "Words tauschen"=1163, "X hoch Y"=1213, "XY-Graph (Klassisch)"=3500, "XY-Graph (Modern)"=21716, "Y-te Wurzel von X"=23062, "Zahl nach boolesches Array"=1814, "Zahl nach Hexadezimal-String"=1181, "Zahl nach Oktal-String"=1182, "Zahl nach String (Dezimaldarstellung)"=1180, "Zahl nach String (Exponentialdarstellung)"=1505, "Zahl nach String (Fließkommadarstellung)"=1506, "Zahl nach String (Technische Notation)"=1183, "Zahl teilen"=1170, "Zahlen verbinden"=1171, "Zeile auswählen"=1510, "Zeilenende-Konstante"=23525, "Zeilenvorschub-Konstante"=23501, "Zeitgesteuerte Schleife"=5570, "Zeitgesteuerte Sequenz"=5573, "Zeitstempel (Blockdiagrammkonstante)"=2068, "Zeitstempel-Anzeigeelement (Klassisch)"=5556, "Zeitstempel-Anzeigeelement (Modern)"=21914, "Zeitstempel-Bedienelement (Klassisch)"=5555, "Zeitstempel-Bedienelement (modern)"=21913, "Zeitstempel-Bedienelement (System)"=21967, "ZerlegenGesperrteDatenWertRef"=2406, "Zufallszahl (0-1)"=1070, "Zugriff verweigern"=8057, "Zugriffsrechte"=1412, "ZusammensetzenSperreAufhebenDatenWertRef (Warnung: gefährlich)"=2407, "Zustand"=2198, "Zustandsdiagramm"=2051, "Öffnen/Erstellen/Ersetzen einer Datei"=8050, "Öffnen/Erstellen/Ersetzen einer Protokolldatei"=8054]
        w64 = refnum<vi> refnum  # NumericConstant
        w52 = refnum<vi> refnum  # SubVI
        w56 = refnum<vi> refnum  # Numeric
        n6 = Open VI Object Reference(7:w56, 8:w48, 10:w45, 11:w40) -> (0:w55:errorcluster, 3:w41:refnum<vi>)
        n7 = property class="Num"(reference=w41, error in=w55) -> (error out=w53:errorcluster, "Terminal"=w49:refnum<vi>)  [unwired: 1 out]
        n8 = New VI Object(vi object class=w52, owner refnum=w47, position/next to=T2 {"Horizontal"=0, "Vertical"=0} ("Position"), 6:w46, 8:w53) -> (object refnum=w82:refnum<vi>, 0:w83:errorcluster)  [unwired: 3 in]
        n9 = New VI Object(vi object class=w70, owner refnum=w47, style=w71, position/next to=T2 {"Horizontal"=0, "Vertical"=0} ("Position"), 8:w83) -> (object refnum=w74:refnum<vi>, 0:w84:errorcluster)  [unwired: 3 in]
        n10 = New VI Object(vi object class=w76, owner refnum=w47, style=w77, position/next to=T2 {"Horizontal"=0, "Vertical"=0} ("Position"), 8:w84) -> (object refnum=w81:refnum<vi>, 0:w85:errorcluster)  [unwired: 3 in]
        n11 = New VI Object(vi object class=w64, owner refnum=w47, style=w65, position/next to=T2 {"Horizontal"=0, "Vertical"=0} ("Position"), 8:w85) -> (object refnum=w68:refnum<vi>, 0:w86:errorcluster)  [unwired: 3 in]
        n12 = property class="NumericConstant"(reference=w81, error in=w86, "Representation"=LVNumericRepresentation."Double Precision" ("Darstellung")) -> (error out=w87:errorcluster)  [unwired: 1 out]
        n13 = property class="NumericConstant"(reference=w68, error in=w87, "Representation"=LVNumericRepresentation."Double Precision" ("Darstellung")) -> (error out=w88:errorcluster)  [unwired: 1 out]
        n14 = property class="SubVI"(reference=w82, error in=w88) -> (error out=w89:errorcluster, "Terms[]"=w63:refnum<vi>[])  [unwired: 1 out]
        n15 = property class="NumericConstant"(reference=w74, error in=w89, "Representation"=LVNumericRepresentation."Double Precision" ("Darstellung")) -> (error out=w90:errorcluster)  [unwired: 1 out]
        n16 = property class="NumericConstant"(reference=w81, error in=w90, "Value"=w44) -> (error out=w91:errorcluster)  [unwired: 1 out]
        n17 = property class="NumericConstant"(reference=w68, error in=w91, "Value"=w43) -> (error out=w92:errorcluster)  [unwired: 1 out]
        n18 = property class="NumericConstant"(reference=w74, error in=w92, "Value"=w42) -> (error out=w93:errorcluster)  [unwired: 1 out]
        n19 = property class="NumericConstant"(reference=w81, error in=w93) -> (error out=w94:errorcluster, "Terminal"=w80:refnum<vi>)  [unwired: 1 out]
        n20 = property class="NumericConstant"(reference=w68, error in=w94) -> (error out=w95:errorcluster, "Terminal"=w69:refnum<vi>)  [unwired: 1 out]
        n21 = property class="NumericConstant"(reference=w74, error in=w95) -> (error out=w96:errorcluster, "Terminal"=w75:refnum<vi>)  [unwired: 1 out]
        n22 = Index Array(array=w63, index=1 ("Index")) -> (element=w61:refnum<vi>)
        n23 = invoke class="Term" method="Verbinden"(reference=w61, error in=w96, "Wire Source"=w80) -> (error out=w97:errorcluster)  [unwired: 4 in, 6 out]
        n24 = Index Array(array=w63, index=3 ("Index")) -> (element=w57:refnum<vi>)
        n25 = invoke class="Term" method="Verbinden"(reference=w57, error in=w97, "Wire Source"=w69) -> (error out=w98:errorcluster)  [unwired: 4 in, 6 out]
        n26 = Index Array(array=w63, index=2 ("Index")) -> (element=w59:refnum<vi>)
        n27 = invoke class="Term" method="Verbinden"(reference=w59, error in=w98, "Wire Source"=w75) -> (error out=w99:errorcluster)  [unwired: 4 in, 6 out]
        n28 = Index Array(array=w63, index=4 ("Index")) -> (element=w50:refnum<vi>)
        n29 = invoke class="Term" method="Verbinden"(reference=w50, error in=w99, "Wire Source"=w49) -> ()  [unwired: 4 in, 7 out]
      }
    }
    n30 = invoke class="Num" method="Löschen"(reference=w26) -> (error out=w35:errorcluster)  [unwired: 2 in, 2 out]
  }
  n31 = invoke class="VI" method="FP.Öffnen"(reference=w3, error in=w10) -> (reference out=w9:refnum<vi>, error out=w8:errorcluster)  [unwired: 3 in, 3 out]
  n32 = property class="VI"(reference=w9, error in=w8) -> (reference out=w12:refnum<vi>, error out=w13:errorcluster, "Diagram"=w14:refnum<vi>)
  n33 = invoke class="TopLvlDiag" method="Bereinigung"(reference=w14, error in=w13) -> (error out=w11:errorcluster)  [unwired: 2 in, 3 out]
  n34 = Close Reference(reference=w12, error in (no error)=w11) -> (error out=w22:errorcluster)
  n35 = call <vilib>:"Simple Error Handler.vi"("error in (no error)"=w22) -> ()  [unwired: 4 in, 5 out]
